vi "WHD_VEten_0.1.4.WS_BIDIR_Cal_05_03_2020.vi"() -> ()   [LabVIEW 2015]
uses:
  <vilib>/LabVIEW Targets/FPGA/cRIO/shared/nicrio_ModuleControls/nicrio_cRIO-9234_DataRatesRing2.ctl
  <vilib>/RTwatchdog.llb/Watchdog expiration actions.ctl
  <vilib>/userdefined/High Color/nirio_resource_hc.ctl
  <vilib>/Platform/TimedLoop/XDataNode/timing_clust.ctl
  <vilib>/Platform/TimedLoop/XDataNode/nitl_modes.ctl
  <vilib>/Platform/TimedLoop/XDataNode/wakeup.ctl
  <vilib>/Analysis/5stat.llb/RMS (DBL).vi
  <vilib>/FPGAPlugInAG/cRIO-9031/niLvFpga_Open_cRIO-9031.vi
  <vilib>/Utility/error.llb/Error Cluster From Error Code.vi
  <vilib>/rvi/errors/niLvFpgaAdjustHostInterfaceError.vi
  <vilib>/FPGAPlugInAG/cRIO-9031/niLvFpga_Run_cRIO-9031.vi
  <vilib>/rvi/interface/common/niFpgaWaitOnOcc.vi
  <vilib>/Utility/file.llb/Write Delimited Spreadsheet (string).vi
  <vilib>/FPGAPlugInAG/cRIO-9031/niLvFpga_Reset_cRIO-9031.vi
  <vilib>/measure/madcrms.llb/Basic Averaged DC-RMS for 1 Chan.vi
  <vilib>/measure/maspectr.llb/FFT Spectrum (Mag-Phase) for 1 Chan.vi
  <vilib>/Utility/config.llb/Write Key (Double).vi
  <vilib>/FPGAPlugInAG/cRIO-9031/niLvFpga_Close_cRIO-9031.vi
  <vilib>/rvi/interface/nirviOpenFPGA/nirviOpenFPGA.xnode
  FPGA Bitfiles/W_RDArabia_FPGATarget_FPGA8a2wsBIdirec_yJvL9yuTbZw.lvbitx
  <vilib>/rvi/interface/nirviReadWriteControl/nirviReadWriteControl.xnode
  <vilib>/rvi/interface/nirviMethod/nirviMethod.xnode
  <vilib>/platform/TimedLoop/XDataNode/XDataNode.xnode
  <vilib>/rvi/interface/nirviCloseFPGA/nirviCloseFPGA.xnode
  <vilib>/NI_Real-Time Target Support.lvlib
  <vilib>/rvi/errors/niLvFpgaMergeErrorWithErrorCode.vi
  AURA_Wheel/Json2Labv.lvlib
  AURA_Wheel/AuraWheelAPI/AuraWheel.lvlib
  NiFpgaLv.dll
  <vilib>/FPGAPlugInAG/cRIO-9031/niLvFpga_ConfigureFifo_cRIO-9031.vi
  <vilib>/FPGAPlugInAG/cRIO-9031/niLvFpga_StartFifo_cRIO-9031.vi
  <vilib>/FPGAPlugInAG/cRIO-9031/niLvFpga_ReadFifo_cRIO-9031.vi
  <vilib>/FPGAPlugInAG/cRIO-9031/niLvFpga_StopFifo_cRIO-9031.vi
  <vilib>/measure/NI_MAPro.lvlib
  <vilib>/Analysis/NI_AALPro.lvlib
  <vilib>/Analysis/NI_AALBase.lvlib
  <vilib>/Utility/config.llb/NI_LVConfig.lvlib
  <vilib>/Platform/TimedLoop/XDataNode/XDNodeRunTimeDep.lvlib
  Library/IF2_Reader/IF2_Reader.lvlib
panel:
  out "T fuera rango":bool
  out "Frequency":dbl[](array[numeric])
  out "Value to compare":dbl[](array[numeric])
  in  "Developer password":string
  out "Waveform Graph":waveform(sgl)[](graph)
  out "min":dbl[](array[numeric])
  out "max":dbl[](array[numeric])
  out "median":dbl[](array[numeric])
  out "mean":dbl[](array[numeric])
  in  "Accelerometer":i32=1 min=1 max=8
  out "Low cutoff freq":dbl
  out "noise_range":dbl
  out "Numeric":i32
  out "Calibration parameter":dbl
  out "Accel.detected":i32
  out "Mean\nfrequency":dbl format="%0.2f"
  out "Nº meas":i32
  out "Array":i32[](array[numeric])
  out "sorted array":i32[](array[numeric])
  out "Array 3":i32[](array[numeric])
  out "max value":i32
  out "max index(es)":i32
  out "element":i32
  out "size(s) 3":i32
  out "size(s)":i32[](array[numeric])
  out "Valid\nindex":i32[](array[numeric])
  out "Acquiring time":dbl
  out "Inicio pasada 2":timestamp
  out "calibration log":path
  out "date/time string 2":string
  out "Folder":path
  in  "Developer commad":string
  out "Save calibration":bool
  out "Pattern amplitude (g)":dbl=1.02
  out "Pattern frequency (Hz)":dbl=159.2
  out "Report":string
  out "AURA wheel test":bool
  out "LOG.txt":path
  out "Report_AURA":string
  out "error FPGA":errorcluster
  out "error AURA":errorcluster
  out "error manipulacion archivos":errorcluster
  out "Response headers":string
  out "Max RMS Ruedas":dbl[][](array[numeric])
  out "TAGs LR6":string[](array[string])
  out "TAGs HEX":string[](array[string])
  out "Parar":bool
  out "result":bool
  out "TAGs":string[](array[string])
  out "Temperatura (ºC)":dbl
  out "V (m/s)":dbl
  out "Digital?":bool=TRUE
  out "Watchdog config":T1={"reset"=FALSE, "occurrence"=FALSE, "trigger protocol"=enum."active high", "trigger line"=enum."none", "disable watchdog on VI exit"=TRUE}
  out "Tiempo de adquisicion":dbl=10.0
  out "Adquirir":bool
  out "Nº Ruedas 1":i32
  out "NºRuedas 2":i32
  out "Disco Duro Disponible (bytes)":i64
  out "Buffer Overflow":bool
  out "Buffer Underflow":bool
  out "Archivo\nvalido?":bool
  out "Número de ejes detectados":i32
  out "Ejes_convoy":i32
  out "Tiempo de paso (s)":dbl
  out "created path":path
  out "Nombre de archivo":path[](array[path])
  out "LR6 IP address":string="192.168.106.94"
  out "Port LR6":u16=2001
  out "Frecuencia de muestreo (Hz)":dbl=25600.0
  out "Escaneos de la FIFO por canal":u32=5000
  out "Tiempo extra al detector de paso (s)":dbl=1.0
  out "dt RMS":dbl=256.0
  out "Frecuencia de muestreo y módulo CRIO":T2=2 items=["51.200 kS/s (NI 9234)"=1, "25.600 kS/s (NI 9234)"=2, "17.067 kS/s (NI 9234)"=3, "12.800 kS/s (NI 9234)"=4, "10.240 kS/s (NI 9234)"=5, "8.533 kS/s (NI 9234)"=6, "7.314 kS/s (NI 9234)"=7, "6.400 kS/s (NI 9234)"=8, "5.689 kS/s (NI 9234)"=9, "5.120 kS/s (NI 9234)"=10, "4.654 kS/s (NI 9234)"=11, "4.267 kS/s (NI 9234)"=12, "3.938 kS/s (NI 9234)"=13, "3.657 kS/s (NI 9234)"=14, "3.413 kS/s (NI 9234)"=15, "3.200 kS/s (NI 9234)"=16, "3.012 kS/s (NI 9234)"=17, "2.845 kS/s (NI 9234)"=18, "2.695 kS/s (NI 9234)"=19, "2.560 kS/s (NI 9234)"=20, "2.438 kS/s (NI 9234)"=21, "2.328 kS/s (NI 9234)"=22, "2.226 kS/s (NI 9234)"=23, "2.133 kS/s (NI 9234)"=24, "2.048 kS/s (NI 9234)"=25, "1.969 kS/s (NI 9234)"=26, "1.896 kS/s (NI 9234)"=27, "1.829 kS/s (NI 9234)"=28, "1.765 kS/s (NI 9234)"=29, "1.707 kS/s (NI 9234)"=30, "1.652 kS/s (NI 9234)"=31]
  out "Puerto RFID":u16=2189
  out "IP RFID":string="192.168.106.99"
  out "Offset_rueda WS 2":fxp<+/-,24,-4>=0.004999998956918716 format="%.27g"
  out "Count(mSec)":u32=2
  out "RFID NEM on?":bool
  out "RFID LR6 on?":bool
  out "Canal cero WS1?":bool
  out "Canal cero WS2":bool
  in  "Calibration":bool
  out "Direccion 0?":bool
  out "Boton Adquirir?":bool
  out "RuedaDetectada2?":bool=TRUE
  out "RuedaDetectada1?":bool=TRUE
  out "Timeout ruedas":dbl
  out "Borrar archivos\nadquisicion con error":bool
  out "Able watchdog?":bool
  out "Reset watchdog?":bool
  out "Leer config RFID NEM":bool
  out "bytes to read":i32
  out "DeviceAddress":u8
  out "timeout ms (60000)":i32
  out "Max archivos":u32=2
  out "Bytes libre despues de borrar":u32=2
  out "Bytes min libre":u32=2
  out "Nº de acelerómetros":i32
  out "Nº inductivos":i32
  out "Offset_rueda WS 1":fxp<+/-,24,-4>=0.004999998956918716 format="%.27g"
  out "TAGs_AURAwheel":string[][](array[string])
  out "Plataformas?":bool
  out "Nº Ejes":i32[](array[numeric])
  out "Nº UTs":i32
  out "it-read-LR6":i32[](array[numeric])
  out "it-LR6":i32
  out "RFID_LR6_Error":errorcluster
  out "Series_flota":string[](array[string])
  out "Tabla_flota":string[][](array[string])
  out "Puntos medios de las ventanas":dbl[][](array[numeric])
  out "configuration file path":path=path "c:/Parametros.cfg"
  out "IP synchr":string
  out "data":cluster{"status":string}
  out "confRFID":path=path "c:/RFID/TAGS.csv"
  out "TAGS leidos":path=path "c:/RFID/TAGS.csv"
  out "Use Aura?":bool
  out "Parametros AuraWheel":string[](array[string])
  out "Parámetros acelerómetros":dbl[](array[numeric])
  out "Fin":bool
  out "Contador":i32=1
  out "Path LOG":path=path "c:/TEST"
  out "Fallo fotocelula":bool
  out "Path_Borrar":path=path "c:/Trenes"
  out "Longitud de la unidad":dbl
  out "Aviso no detección":string
  out "Time to Acquire Block (ms)":i32
  out "Distancia de acelerómetros":dbl[](array[numeric])
  out "Block Size":u32
  out "Distancias generales":dbl[](array[numeric])
  out "Reset del controlador":bool
  out "Parar la aplicación":bool
  out "date/time string":string
  out "Timeout ruedas":bool
  out "Tiempo":dbl
  out "Inicio pasada":timestamp
  out "Ultimo TEST":timestamp
  out "Fuente":bool=TRUE
  out "DC OK":string
  out "Aviso temperatura":string
  out "connection ID":refnum<k5>
  # "Calibration - Noise analysis"
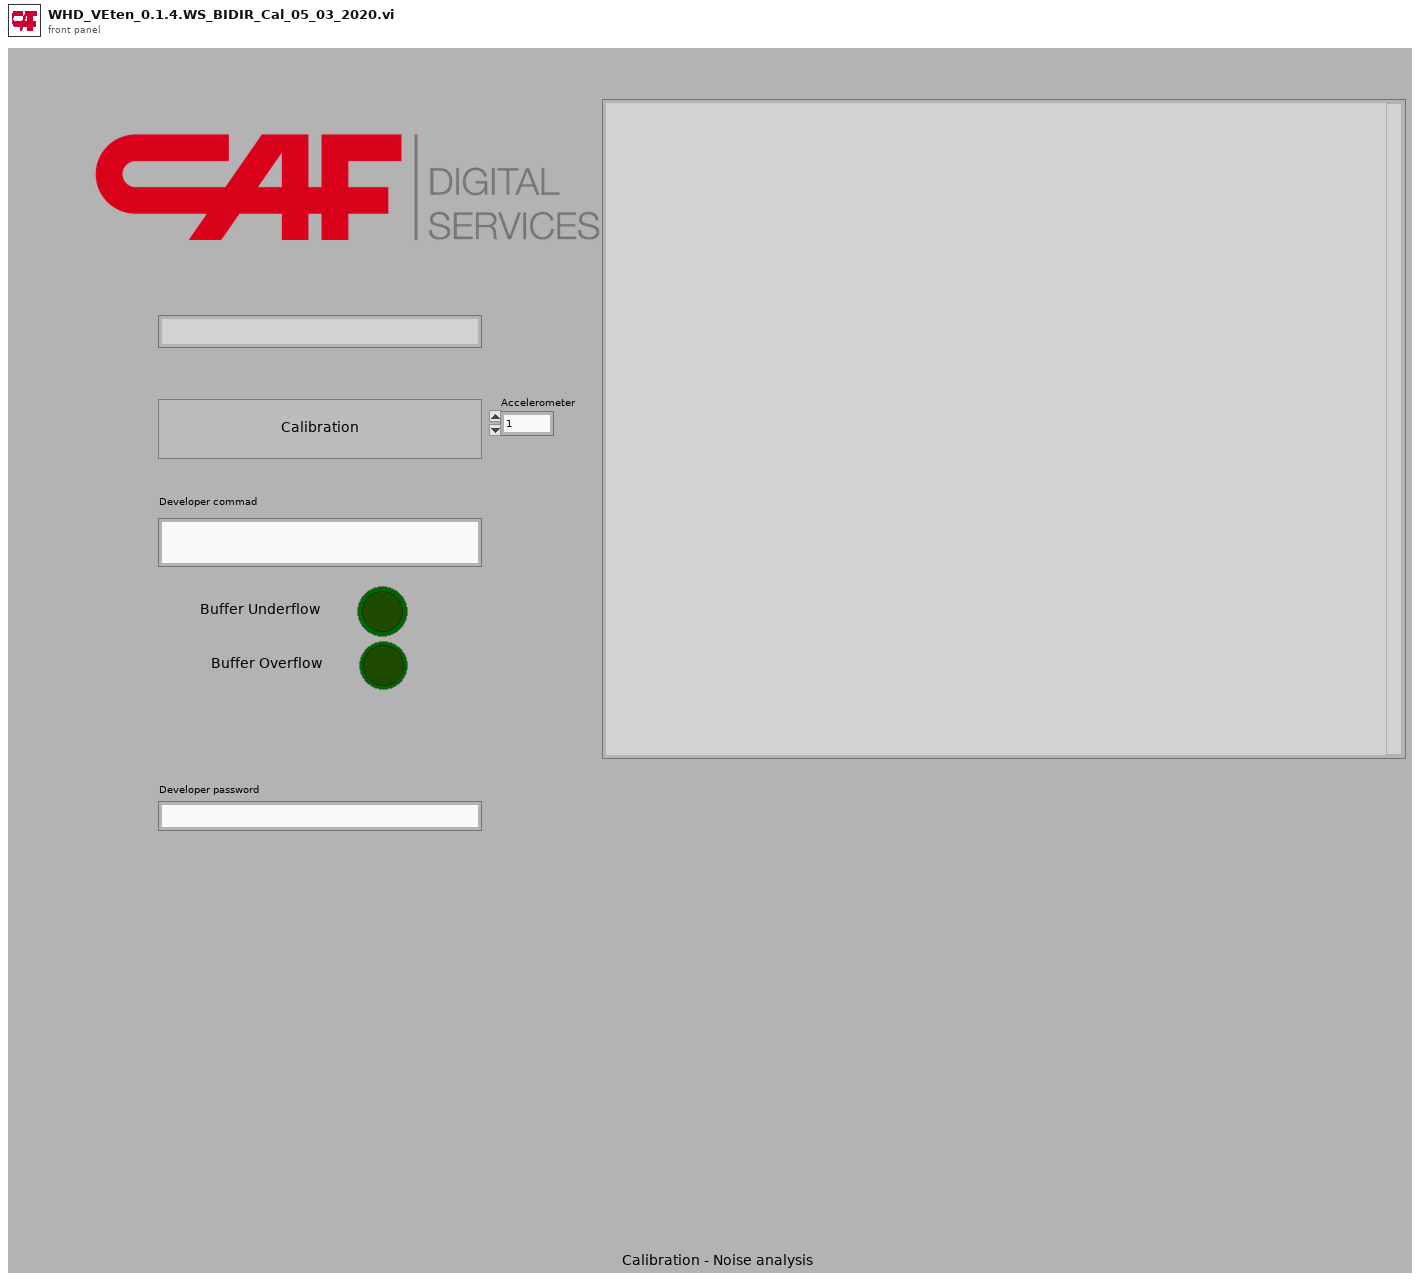
[diagram p1: front panel]
types:
  T1 = typedef "Watchdog expiration actions.ctl" = cluster{"reset":bool, "occurrence":bool, "trigger protocol":enum16{"active high", "active low", "open collector"}, "trigger line":enum16{"none", "line 0", "line 1", "line 2", "line 3", "line 4", "line 5", "line 6", "line 7", "SMB line 0"}, "disable watchdog on VI exit":bool}
  T2 = typedef "nicrio_cRIO-9234_DataRatesRing2.ctl" = u8
  T3 = typedef "nirio_resource_hc.ctl" = tag
  T4 = enum16{"open", "replace", "create", "open or create", "replace or create", "replace or create with confirmation"}
  T5 = enum16{"big-endian, network order", "native, host order", "little-endian"}
  T6 = typedef "XDNodeRunTimeDep.lvlib/timing_clust.ctl" = cluster{"Expected End [f-1]":u64, "Actual End [f-1]":u64, "Finished Late? [f-1]":bool, "Expected End [i-1]":u64, "Actual End [i-1]":u64, "Finished Late? [i-1]":bool, "Expected Start [i]":u64, "Actual Start [i]":u64, "Expected Start [f]":u64, "Actual Start [f]":u64, "Source Name":string, "Structure Name":string, "Period":i64, "Deadline":i64, "Offset":i64, "Start":i64, "Priority":i32, "Timeout":i32, "Mode":T7, "Wakeup Reason":T8, "Error":errorcluster, "Source Type":string, "Secondary Source Type":string, "Global End Time":u64, "Global Start Time":u64, "Frame Duration":u64, "Iteration Duration":u64, "Assigned CPU":i32, "I/O Scan Engine Mode":u32}
  T7 = typedef "XDNodeRunTimeDep.lvlib/nitl_modes.ctl" = enum32{"No Change", "Process missed periods, maintain original phase", "Discard missed periods, maintain original phase", "Process missed periods, ignore original phase", "Discard missed periods, ignore original phase"}
  T8 = typedef "XDNodeRunTimeDep.lvlib/wakeup.ctl" = enum32{"Normal", "Aborted", "Asynchronous wakeup", "Timing source error", "Timed loop error", "Timeout"}
  T9 = cluster{"error IO":errorcluster, bool[], u32[], string[], dbl[]}
  T10 = cluster{"error out":errorcluster, dbl[], "Normalized Tags":string[], "Direccion 0?":bool}
  T11 = cluster{"g_ts":dbl, "p_sp":dbl, "p_tp":dbl, "p_tg":cluster{"tg_n":dbl, "tg_t":string}[], "p_ax":cluster{"ax_n":dbl, "ax_sp":dbl, "ax_wh":cluster{"wh_p":dbl, "wh_a1":dbl, "wh_a2":dbl, "wh_a3":dbl, "wh_a4":dbl}[]}[]}
  T12 = typedef "NI_LVConfig.lvlib/Config Data RefNum.ctl" = refnum<k1>
  T13 = cluster{"IP":string, "Port":u16, "ReaderConfigFile":path, "ROspecConfigFile":path}
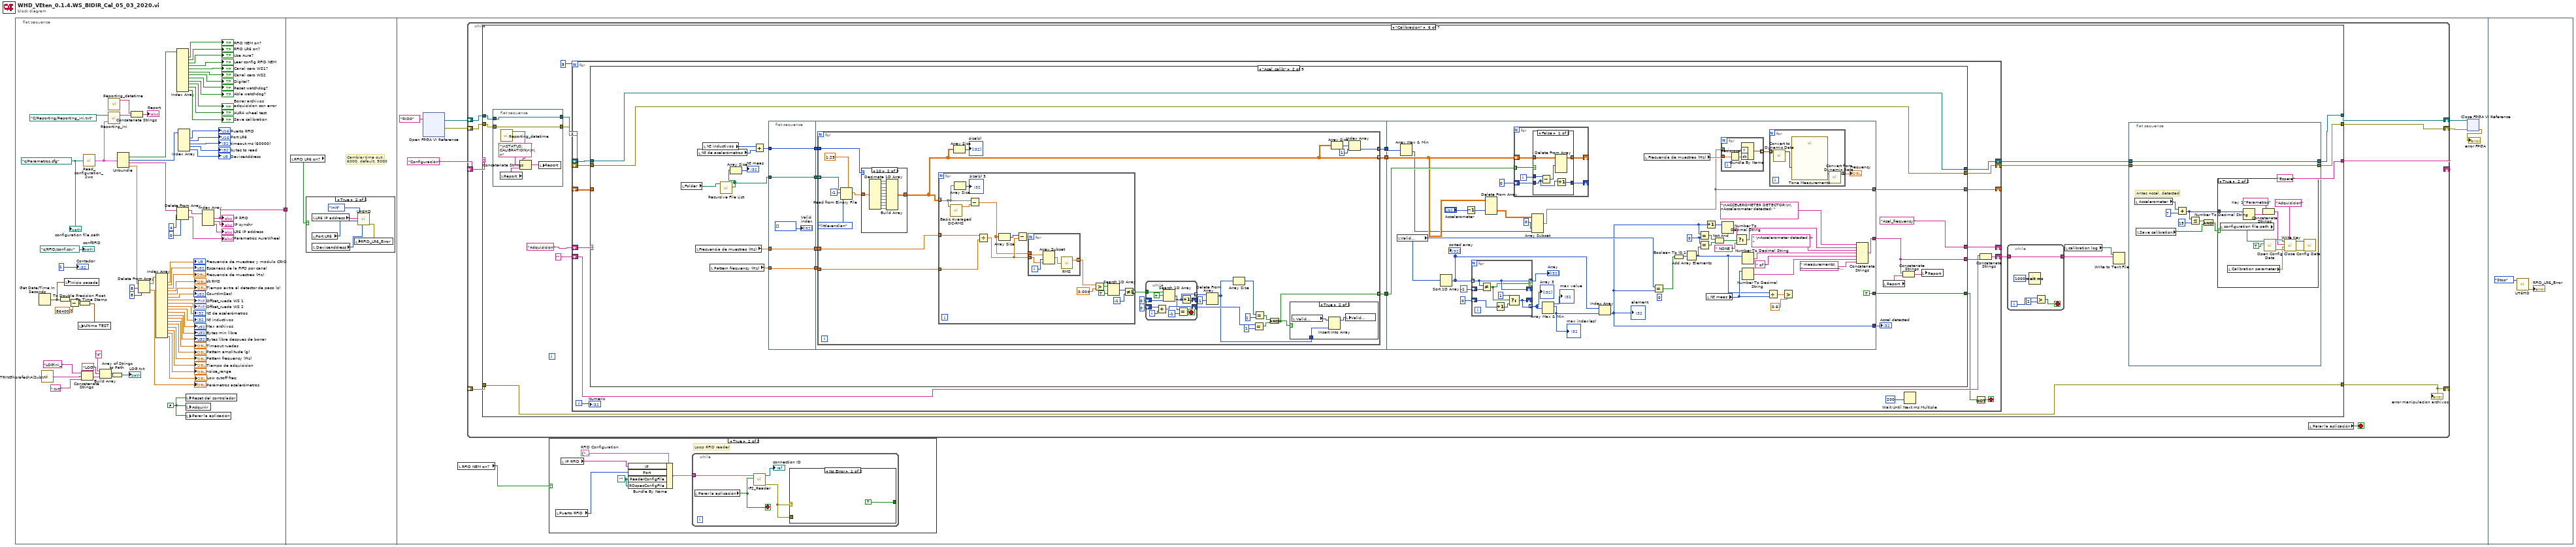
[diagram p0: block diagram]
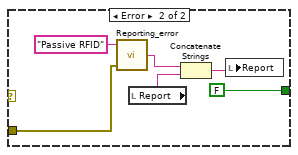
[diagram p4: hidden frame]
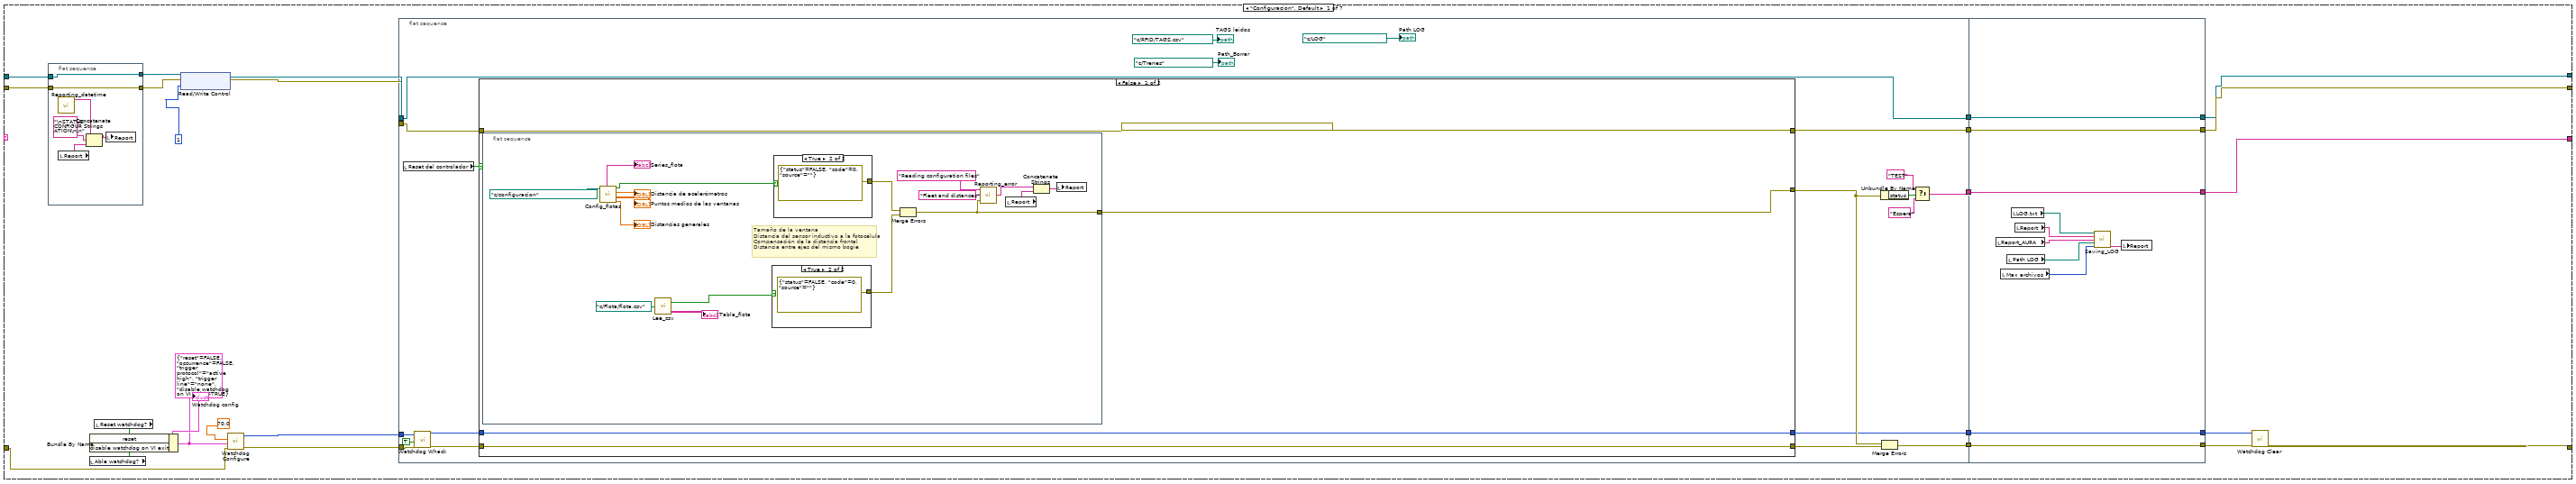
[diagram p5: hidden frame]
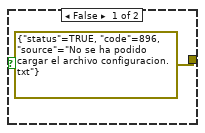
[diagram p6: hidden frame]
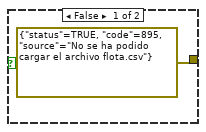
[diagram p7: hidden frame]
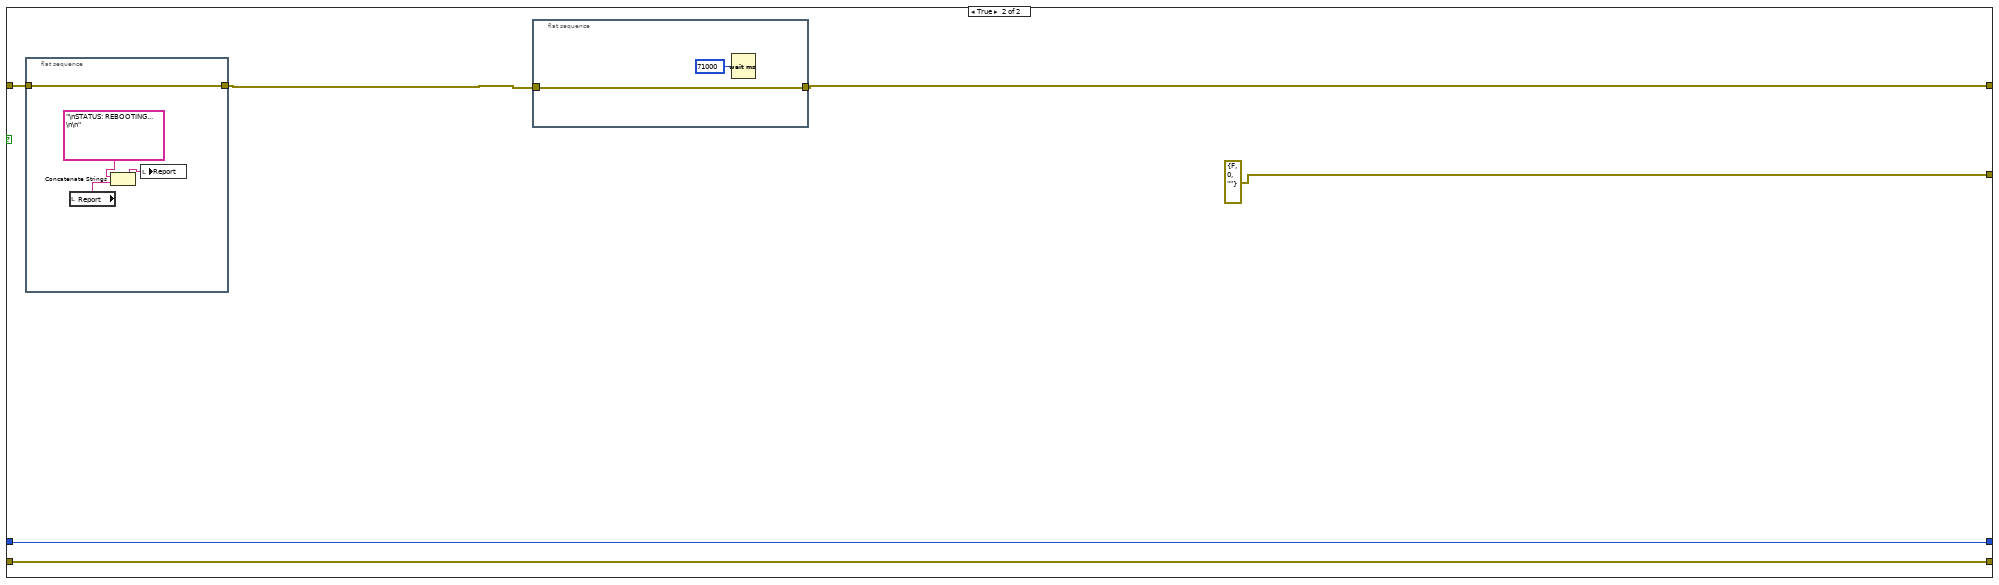
[diagram p8: hidden frame]
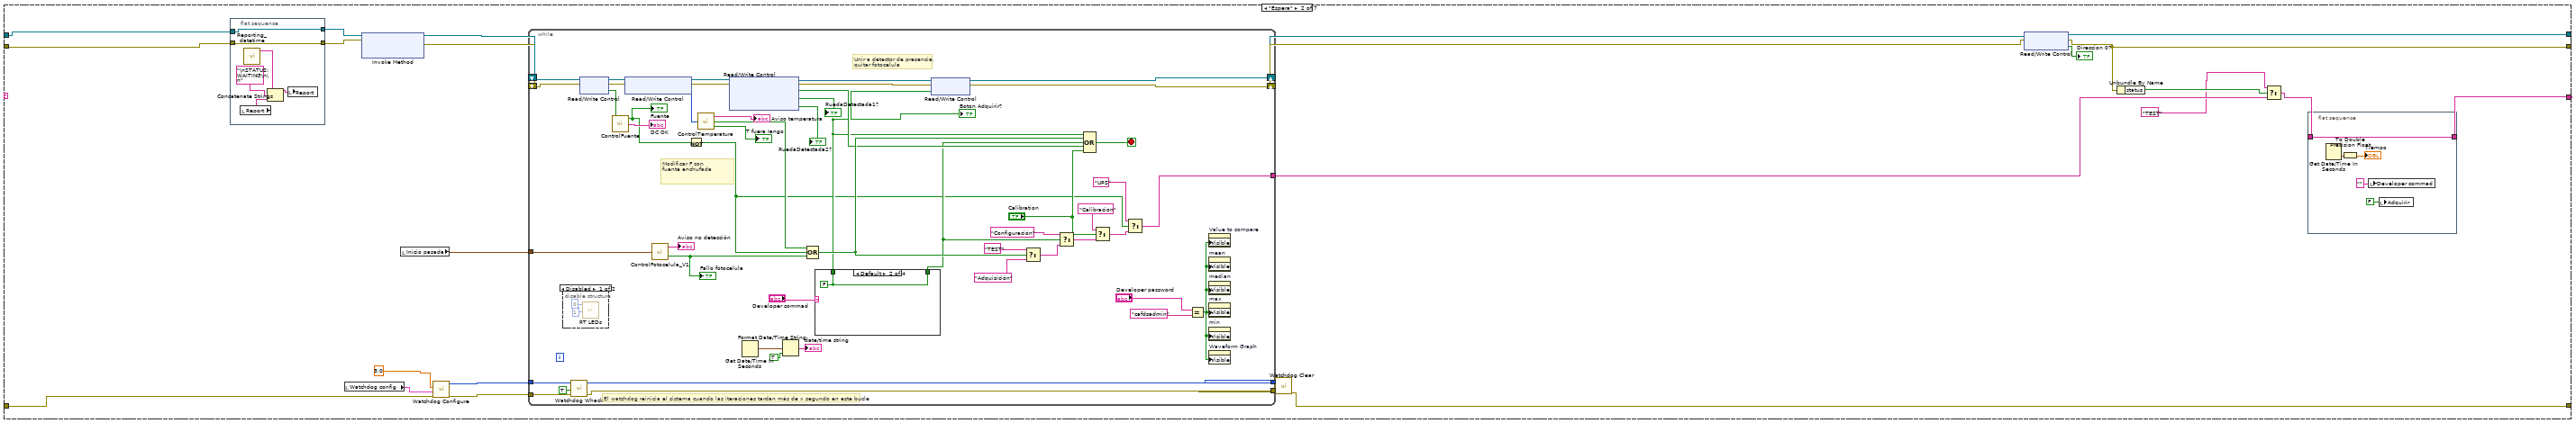
[diagram p9: hidden frame]
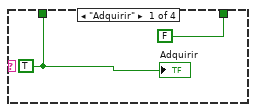
[diagram p10: hidden frame]
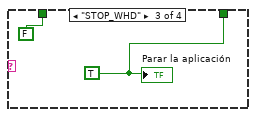
[diagram p11: hidden frame]
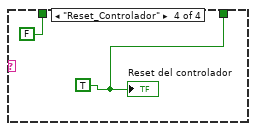
[diagram p12: hidden frame]
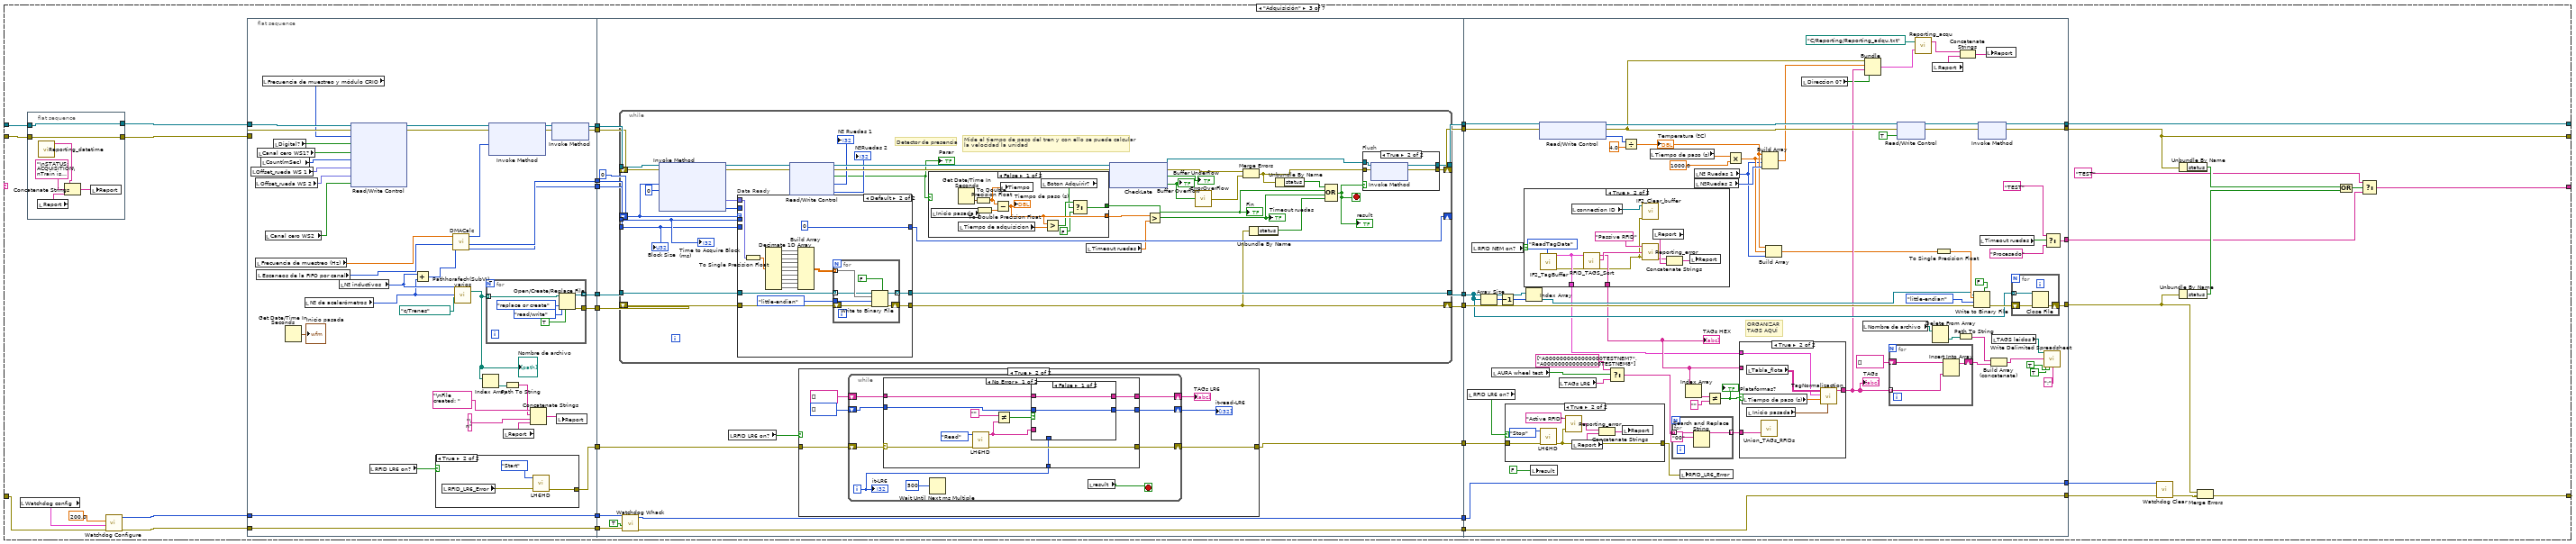
[diagram p14: hidden frame]
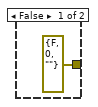
[diagram p15: hidden frame]
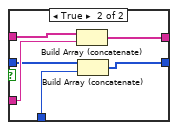
[diagram p17: hidden frame]
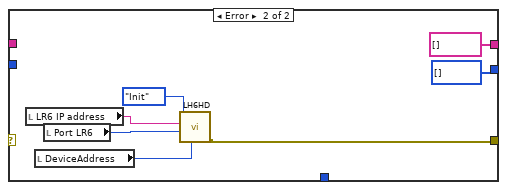
[diagram p18: hidden frame]
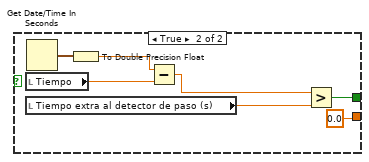
[diagram p19: hidden frame]
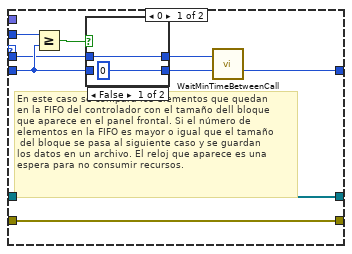
[diagram p20: hidden frame]
diagram:
  n1 = flat-sequence {
    tunnel: [w4] -> w1
    tunnel: w1 -> [_]
    frame #0 {
      w5 = FALSE ("Reset del controlador")
      w66 = path "c:/Parametros.cfg" ("configuration file path")
      n2 = Get Date/Time In Seconds() -> (seconds since 1Jan1904=w71:timestamp)
      n3 = call "STRINGhorafechA(SubVI).vi"() -> ("STRINGhora_fecha"=w16:string)
      n4 = To Double Precision Float(number=w71) -> (double precision float=w73:dbl)
      n5 = local write "Inicio pasada"(w71) -> ()
      n6 = Subtract(x=w73, y=86400.0) -> (x-y=w72:dbl)
      n7 = To Time Stamp(1:w72) -> (0:w70:timestamp)
      n8 = local write "Ultimo TEST"(w70) -> ()
      n9 = Concatenate Strings("LOGini_" ("string"), w16, ".txt" ("string")) -> (w18:string)
      n10 = call "Read_configuration_2ws.vi"("configuration file path"=w66) -> ("output cluster"=w22:T9)
      n11 = Build Array("c", "LOG" ("element"), w18) -> (w15:string[])
      n12 = call "Reporting_ini.vi"("Configuration cluster"=w22, "address repoting"=path "C:/Reporting/Reporting_ini.txt" ("file (use dialog)")) -> ("Reporting"=w21:string)  [unwired: 1 in]
      n13 = call "Reporting_datetime.vi"() -> ("String"=w19:string)  [unwired: 11 in]
      n14 = Array of Strings to Path(0:w15) -> (2:→"LOG.txt":path)  [unwired: 1 out]
      n15 = Unbundle(w22) -> (w69:bool[], w68:u32[], w61:string[], w65:dbl[])  [unwired: 1 out]
      n16 = Concatenate Strings(w19, w21) -> (→"Report":string)
      n17 = Delete From Array(array=w65, length=8, index=8) -> (deleted portion=→"Parámetros acelerómetros":dbl[], array with subset deleted=w64:dbl[])
      n18 = Index Array(array=w64) -> (element #1=→"Frecuencia de muestreo y módulo CRIO":dbl, element #2=→"Escaneos de la FIFO por canal":dbl, element #3=→"Frecuencia de muestreo (Hz)":dbl, element #4=→"dt RMS":dbl, element #5=→"Tiempo extra al detector de paso (s)":dbl, element #6=→"Count(mSec)":dbl, element #7=→"Offset_rueda WS 1":dbl, element #8=→"Offset_rueda WS 2":dbl, element #9=→"Nº de acelerómetros":dbl, element #10=→"Nº inductivos":dbl, element #11=→"Max archivos":dbl, element #12=→"Bytes min libre":dbl, element #13=→"Bytes libre despues de borrar":dbl, element #14=→"Timeout ruedas":dbl, element #15=→"Pattern amplitude (g)":dbl, element #16=→"Pattern frequency (Hz)":dbl, element #17=→"Tiempo de adquisicion":dbl, element #18=→"noise_range":dbl, element #19=→"Low cutoff freq":dbl)  [unwired: 19 in]
      n19 = Index Array(array=w69) -> (element #1=→"RFID NEM on?":bool, element #2=→"RFID LR6 on?":bool, element #3=→"Use Aura?":bool, element #4=→"Leer config RFID NEM":bool, element #5=→"Canal cero WS1?":bool, element #6=→"Canal cero WS2":bool, element #7=→"Digital?":bool, element #8=→"Reset watchdog?":bool, element #9=→"Able watchdog?":bool, element #10=→"Borrar archivos\nadquisicion con error":bool, element #11=→"AURA wheel test":bool, element #12=→"Save calibration":bool)  [unwired: 12 in]
      n20 = Delete From Array(array=w61, length=4, index=0) -> (deleted portion=→"Parametros AuraWheel":string[], array with subset deleted=w60:string[])
      n21 = Index Array(array=w68) -> (element #1=→"Puerto RFID":u32, element #2=→"Port LR6":u32, element #3=→"timeout ms (60000)":u32, element #4=→"bytes to read":u32, element #5=→"DeviceAddress":u32)  [unwired: 5 in]
      n22 = local write "Reset del controlador"(w5) -> ()
      n23 = local write "Adquirir"(w5) -> ()
      n24 = local write "Parar la aplicación"(w5) -> ()
      n25 = Index Array(array=w60) -> (element #1=w4:string, element #2=→"IP synchr":string, element #3=→"LR6 IP address":string)  [unwired: 3 in]
      "IP RFID" <- w4
      "Contador" <- 1
      "confRFID" <- path "c:/RFID/conf.csv" ("file path (use dialog)")
      "configuration file path" <- w66
    }
    frame #1 {
      # "Cambiar time out:\n6000, default, 5000"
      n26 = local read "RFID LR6 on?"() -> (w75:bool)
      n27 = case shown="True" w75 {
        frame False {
        }
        frame True {
          n28 = local read "LR6 IP address"() -> (w76:string)
          n29 = local read "Port LR6"() -> (w77:u16)
          n30 = local read "DeviceAddress"() -> (w78:u8)
          n31 = call "LH6HD.vi"("DeviceAddress"=w78, "Reader Port"=w77, "IP Address"=w76, "Action"=enum16{"Init", "Start", "Read", "Stop", "Exit"}."Init") -> ("error out"=w80:errorcluster)  [unwired: 6 in, 1 out]
          n32 = local write "RFID_LR6_Error"(w80) -> ()
        }
      }
    }
    frame #2 {
      n33 = xnode "Open FPGA VI Reference"("resource name"=T3 "RIO0") -> ("FPGA VI Reference Out"=w88:refnum<k20>, "error out"=w87:errorcluster)  [unwired: 1 in]
      n34 = local read "RFID NEM on?"() -> (w81:bool)
      n35 = while {
        shift-right: [w105] -> _
        shift-left: "Configuración" -> [w113]
        shift-right: [w107] -> w84
        shift-left: w88 -> [w112]
        shift-right: [w106] -> w83
        shift-left: w87 -> [w111]
        shift-right: [w110] -> _
        shift-left: _ -> [w109]
        stop <- w108 stop-if-true
        n36 = case shown="\"Calibracion\"" w113 {
          tunnel: [w128 w231 w326 w676 w924 "Espera" "Espera" ("t")] -> w105
          tunnel: [w138 w219 w340 w665 w923 w992 w1791] -> w107
          tunnel: [w139 w218 w341 w663 w922 w990 w1790] -> w106
          tunnel: w112 -> [w122 w217 w312 w666 w923 w1002 w1793]
          tunnel: w111 -> [w121 w216 w311 w664 w915 w1001 w1792]
          tunnel: [w135 w225 w338 w661 w914 w991 w1788] -> w110
          tunnel: w109 -> [w127 w230 w322 w675 w911 w991 w1788]
          frame "Configuración", Default {
            n37 = flat-sequence {
              tunnel: w122 -> [w145]
              tunnel: w121 -> [w144]
              tunnel: [w145] -> w120
              tunnel: [w144] -> w119
              frame #0 {
                n38 = call "Reporting_datetime.vi"() -> ("String"=w140:string)  [unwired: 11 in]
                n39 = local read "Report"() -> (w141:string)
                n40 = Concatenate Strings(w140, "\nSTATUS: CONFIGURATION\n\n", w141) -> (w143:string)
                n41 = local write "Report"(w143) -> ()
              }
            }
            n42 = local read "Able watchdog?"() -> (w132:bool)
            n43 = local read "Reset watchdog?"() -> (w133:bool)
            n44 = Bundle By Name(cluster=T1 {"reset"=FALSE, "occurrence"=FALSE, "trigger protocol"=enum."active high", "trigger line"=enum."none", "disable watchdog on VI exit"=TRUE} ("expiration actions"), "reset"=w133, "disable watchdog on VI exit"=w132) -> (w126:T1)
            "Watchdog config" <- w126
            n45 = xnode "Read/Write Control"("FPGA VI Reference In"=w120, "error in"=w119, "Cycles to Filter"=u16 1) -> ("FPGA VI Reference Out"=w131:refnum<k20>, "error out"=w130:errorcluster)
            n46 = call <vilib>:"Watchdog Configure.vi"("error in (no error)"=w127, "expiration actions"=w126, "timeout (1 sec)"=70.0) -> ("error out"=w123:errorcluster, "watchdogID"=w124:u64)  [unwired: 1 in, 2 out]
            n47 = flat-sequence {
              tunnel: w131 -> [w157]
              tunnel: w130 -> [w154]
              tunnel: w124 -> [w147]
              tunnel: w123 -> [w146]
              tunnel: [w156] -> w118
              tunnel: [w164] -> w117
              tunnel: [w157] -> w116
              tunnel: [w159] -> w115
              tunnel: [w151] -> w114
              tunnel: [w209] -> w137
              tunnel: [w210] -> w136
              tunnel: [w211] -> w138
              tunnel: [w212] -> w128
              tunnel: [w213] -> w139
              tunnel: w118 -> [w213]
              tunnel: w117 -> [w212]
              tunnel: w116 -> [w211]
              tunnel: w115 -> [w210]
              tunnel: w114 -> [w209]
              frame #0 {
                n48 = local read "Reset del controlador"() -> (w153:bool)
                n49 = call <vilib>:"Watchdog Whack.vi"("error in (no error)"=w146, "reset watchdog after expire? (F)"=TRUE, "watchdogID in"=w147) -> ("error out"=w149:errorcluster, "watchdogID out"=w150:u64)  [unwired: 2 in, 1 out]
                n50 = case shown="False" w153 {
                  tunnel: w154 -> [w169 w192]
                  tunnel: [w169 w195] -> w156
                  tunnel: [w166 errorcluster {"status"=FALSE, "code"=0, "source"=""} ("error IO")] -> w155
                  tunnel: [w168 w194] -> w151
                  tunnel: w150 -> [w168 w194]
                  tunnel: w149 -> [w167 w193]
                  tunnel: [w167 w193] -> w148
                  frame False {
                    n51 = flat-sequence {
                      tunnel: [w170] -> w166
                      frame #0 {
                        # "Tamaño de la ventana\nDistancia del sensor inductivo a la fotocélula\nCompensación de la distancia frontal\nDistancia entre ejes del mismo bogie"
                        n52 = call "Config_flotas.vi"("file path (dialog if empty)"=path "c:/configuracion") -> ("Distancias generales"=→"Distancias generales":dbl[], "Puntos medios de las ventanas"=→"Puntos medios de las ventanas":dbl[][], "Distancia de acelerómetros"=→"Distancia de acelerómetros":dbl[], "Distacias y medidas de dispositivos"=w183:bool, "Series_flota"=→"Series_flota":string[])  [unwired: 3 in]
                        n53 = call "Lee_csv.vi"("Path"=path "c:/Flota/flota.csv") -> ("Tabla_flota"=→"Tabla_flota":string[][], "Lectura_OK?"=w180:bool)
                        n54 = case shown="True" w180 {
                          tunnel: [errorcluster {"status"=TRUE, "code"=895, "source"="No se ha podido cargar el archivo flota.csv"} ("error out") errorcluster {"status"=FALSE, "code"=0, "source"=""} ("error out")] -> w184
                          frame False {
                          }
                          frame True {
                          }
                        }
                        n55 = case shown="True" w183 {
                          tunnel: [errorcluster {"status"=TRUE, "code"=896, "source"="No se ha podido cargar el archivo configuracion.txt"} ("error out") errorcluster {"status"=FALSE, "code"=0, "source"=""} ("error out")] -> w185
                          frame False {
                          }
                          frame True {
                          }
                        }
                        n56 = Merge Errors(w185, w184) -> (w170:errorcluster)
                        n57 = call "Reporting_error.vi"("error out 2"=w170, "Concept explanation"="Fleet and distances", "Concept"="Reading configuration files") -> ("Reporting"=w172:string)
                        n58 = local read "Report"() -> (w171:string)
                        n59 = Concatenate Strings(w172, w171) -> (w173:string)
                        n60 = local write "Report"(w173) -> ()
                      }
                    }
                  }
                  frame True {
                    n61 = flat-sequence {
                      tunnel: w192 -> [w200]
                      tunnel: [w200] -> w191
                      frame #0 {
                        n62 = local read "Report"() -> (w199:string)
                        n63 = Concatenate Strings("\nSTATUS: REBOOTING...\n\n", w199) -> (w197:string)
                        n64 = local write "Report"(w197) -> ()
                      }
                    }
                    n65 = flat-sequence {
                      tunnel: [w202] -> w195
                      tunnel: w191 -> [w202]
                      frame #0 {
                        n66 = Wait (ms)(milliseconds to wait=u32 71000) -> ()  [unwired: 1 out]
                      }
                    }
                  }
                }
                n67 = Unbundle By Name(w155) -> ("status"=w165:bool)
                n68 = Merge Errors(w155, w148) -> (w159:errorcluster)
                n69 = Select(t="TEST", s=w165, f="Espera") -> (s? t:f=w164:string)
                "Path_Borrar" <- path "c:/Trenes" ("file path (use dialog)")
                "Path LOG" <- path "c:/LOG" ("file path (use dialog)")
                "TAGS leidos" <- path "c:/RFID/TAGS.csv" ("file path (use dialog)")
              }
              frame #1 {
                n70 = local read "Report_AURA"() -> (w206:string)
                n71 = local read "Max archivos"() -> (w207:u32)
                n72 = local read "Path LOG"() -> (w208:path)
                n73 = local read "LOG.txt"() -> (w203:path)
                n74 = local read "Report"() -> (w205:string)
                n75 = call "Saving_LOG.vi"("Path"=w203, "Report"=w205, "Report AURA"=w206, "Path Carpeta"=w208, "Nº Archivos Max"=w207) -> ("Report"=w204:string)  [unwired: 9 in, 1 out]
                n76 = local write "Report"(w204) -> ()
              }
            }
            n77 = call <vilib>:"Watchdog Clear.vi"("error in (no error)"=w136, "watchdogID in"=w137) -> ("error out"=w135:errorcluster)  [unwired: 5 in]
          }
          frame "Espera" {
            n78 = flat-sequence {
              tunnel: w217 -> [w244]
              tunnel: w216 -> [w243]
              tunnel: [w244] -> w215
              tunnel: [w243] -> w214
              frame #0 {
                n79 = local read "Report"() -> (w240:string)
                n80 = call "Reporting_datetime.vi"() -> ("String"=w239:string)  [unwired: 11 in]
                n81 = Concatenate Strings(w239, "\nSTATUS: WAITING\n\n", w240) -> (w242:string)
                n82 = local write "Report"(w242) -> ()
              }
            }
            n83 = local read "Watchdog config"() -> (w224:T1)
            n84 = xnode "Invoke Method"("FPGA VI Reference In"=w215, "error in"=w214) -> ("FPGA VI Reference Out"=w234:refnum<k20>, "error out"=w233:errorcluster)  [unwired: 1 in]
            n85 = local read "Inicio pasada"() -> (w238:timestamp)
            n86 = call <vilib>:"Watchdog Configure.vi"("error in (no error)"=w230, "expiration actions"=w224, "timeout (1 sec)"=3.0) -> ("error out"=w229:errorcluster, "watchdogID"=w228:u64)  [unwired: 1 in, 2 out]
            n87 = while {
              tunnel: [w255] -> w237
              shift-right: [w271] -> w220
              shift-left: w234 -> [w279]
              shift-right: [w270] -> w221
              shift-left: w233 -> [w278]
              tunnel: w238 -> [w282]
              tunnel: w229 -> [w268]
              tunnel: w228 -> [w269]
              tunnel: [w267] -> w227
              tunnel: [w266] -> w226
              stop <- w261 stop-if-true
              # "Modificar F con\nfuente enchufada"
              # "Unir a detector de presencia,\nquitar fotocelula"
              # "El watchdog reinicia el sistema cuando las iteraciones tardan más de x segundo en este bucle"
              n88 = disable-structure shown="Disabled" {
                frame Disabled {
                  n89 = call <vilib>:"RT LEDs.vi"("State"=1, "LED Num"=0) -> ()  [unwired: 1 in, 5 out]
                }
                frame Enabled {
                }
              }
              n90 = call <vilib>:"Watchdog Whack.vi"("error in (no error)"=w268, "reset watchdog after expire? (F)"=TRUE, "watchdogID in"=w269) -> ("error out"=w266:errorcluster, "watchdogID out"=w267:u64)  [unwired: 2 in, 1 out]
              n91 = xnode "Read/Write Control"("FPGA VI Reference In"=w279, "error in"=w278) -> ("FPGA VI Reference Out"=w291:refnum<k20>, "error out"=w290:errorcluster, "DC OK"=w295:bool)
              n92 = call "ControlFuente.vi"("DC OK 3"=w295) -> ("DC OK 2"=w257:bool, "DC OK"=→"DC OK":string)  [unwired: 1 out]
              "Fuente" <- w257
              n93 = xnode "Read/Write Control"("FPGA VI Reference In"=w291, "error in"=w290) -> ("FPGA VI Reference Out"=w286:refnum<k20>, "error out"=w285:errorcluster, "Chassis Temperature"=w293:i16)
              n94 = call "ControlFotocelula_V1.vi"("Tiempo de entrada a espera"=w282) -> ("Aviso no detección"=→"Aviso no detección":string, "Boolean"=w283:bool)
              "Fallo fotocelula" <- w283
              n95 = Not(x=w257) -> (.not. x?=w253:bool)
              n96 = call "ControlTemperatura.vi"("Chassis Temperature"=w293) -> ("Aviso temperatura"=→"Aviso temperatura":string, "Boolean"=w287:bool, "T fuera rango"=→"T fuera rango":bool)
              n97 = xnode "Read/Write Control"("FPGA VI Reference In"=w286, "error in"=w285) -> ("FPGA VI Reference Out"=w281:refnum<k20>, "error out"=w280:errorcluster, "Detector de presencia"=w274:bool, "RuedaDetectada1?"=→"RuedaDetectada1?":bool, "RuedaDetectada2?"=→"RuedaDetectada2?":bool)
              n98 = Get Date/Time In Seconds() -> (seconds since 1Jan1904=w276:timestamp)
              n99 = Format Date/Time String(seconds (now)=w276, UTC format=TRUE) -> (date/time string=→"date/time string":string)  [unwired: 1 in]
              n100 = Compound Arithmetic op=OR(w287, w253, w283) -> (w284:bool)
              n101 = case shown="Default" "Developer commad" {
                tunnel: [w301 w302 FALSE ("Adquirir") FALSE ("Adquirir")] -> w260
                tunnel: [FALSE ("Adquirir") w302 w303 w305] -> w259
                frame "Adquirir" {
                  w301 = TRUE ("Adquirir")
                  "Adquirir" <- w301
                }
                frame Default {
                  w302 = FALSE ("Adquirir")
                }
                frame "STOP_WHD" {
                  w303 = TRUE ("Adquirir")
                  "Parar la aplicación" <- w303
                }
                frame "Reset_Controlador" {
                  w305 = TRUE ("Adquirir")
                  "Reset del controlador" <- w305
                }
              }
              "Boton Adquirir?" <- w260
              n102 = xnode "Read/Write Control"("FPGA VI Reference In"=w281, "error in"=w280, "Fotocélula"=w260) -> ("FPGA VI Reference Out"=w271:refnum<k20>, "error out"=w270:errorcluster)
              n103 = Select(t="TEST", s=w284, f="Adquisición") -> (s? t:f=w296:string)
              n104 = Select(t="Configuración", s=w259, f=w296) -> (s? t:f=w264:string)
              n105 = Compound Arithmetic op=OR(w260, w284, w259, w274, "Calibration") -> (w261:bool)
              n106 = Select(t="Calibracion", s="Calibration", f=w264) -> (s? t:f=w256:string)
              n107 = Select(t="UPS", s=w253, f=w256) -> (s? t:f=w255:string)
              n108 = Equal?(x="Developer password", y="cafdsadmin") -> (x = y?=w250:bool)
              n109 = property on="Value to compare" class="Arr (strict)"("Visible"=w250) -> ()  [unwired: 2 in, 2 out]
              n110 = property on="mean" class="Arr (strict)"("Visible"=w250) -> ()  [unwired: 2 in, 2 out]
              n111 = property on="median" class="Arr (strict)"("Visible"=w250) -> ()  [unwired: 2 in, 2 out]
              n112 = property on="max" class="Arr (strict)"("Visible"=w250) -> ()  [unwired: 2 in, 2 out]
              n113 = property on="min" class="Arr (strict)"("Visible"=w250) -> ()  [unwired: 2 in, 2 out]
              n114 = property on="Waveform Graph" class="WFGraph (strict)"("Visible"=w250) -> ()  [unwired: 2 in, 2 out]
            }
            n115 = call <vilib>:"Watchdog Clear.vi"("error in (no error)"=w226, "watchdogID in"=w227) -> ("error out"=w225:errorcluster)  [unwired: 5 in]
            n116 = xnode "Read/Write Control"("FPGA VI Reference In"=w220, "error in"=w221) -> ("FPGA VI Reference Out"=w219:refnum<k20>, "error out"=w218:errorcluster, "Direccion 0?"=→"Direccion 0?":bool)
            n117 = Unbundle By Name(w218) -> ("status"=w236:bool)
            n118 = Select(t="TEST", s=w236, f=w237) -> (s? t:f=w232:string)
            n119 = flat-sequence {
              tunnel: [w248] -> w231
              tunnel: w232 -> [w248]
              frame #0 {
                n120 = Get Date/Time In Seconds() -> (seconds since 1Jan1904=w249:timestamp)
                n121 = To Double Precision Float(number=w249) -> (double precision float=→"Tiempo":dbl)
                n122 = local write "Developer commad"("" ("Developer commad")) -> ()
                n123 = local write "Adquirir"(FALSE ("Adquirir")) -> ()
              }
            }
          }
          frame "Adquisición" {
            n124 = local read "Watchdog config"() -> (w323:T1)
            n125 = flat-sequence {
              tunnel: w312 -> [w352]
              tunnel: w311 -> [w351]
              tunnel: [w352] -> w310
              tunnel: [w351] -> w309
              frame #0 {
                n126 = local read "Report"() -> (w348:string)
                n127 = call "Reporting_datetime.vi"() -> ("String"=w347:string)  [unwired: 11 in]
                n128 = Concatenate Strings(w347, "\nSTATUS: ACQUISITION\nTrain is passing\n\n", w348) -> (w350:string)
                n129 = local write "Report"(w350) -> ()
              }
            }
            n130 = call <vilib>:"Watchdog Configure.vi"("error in (no error)"=w322, "expiration actions"=w323, "timeout (1 sec)"=200.0) -> ("error out"=w320:errorcluster, "watchdogID"=w321:u64)  [unwired: 1 in, 2 out]
            n131 = flat-sequence {
              tunnel: w309 -> [w386]
              tunnel: w310 -> [w387]
              tunnel: [w385] -> w337
              tunnel: [w384] -> w336
              tunnel: [w383] -> w335
              tunnel: [w382] -> w334
              tunnel: [w381] -> w333
              tunnel: [w380] -> w332
              tunnel: [w370] -> w325
              tunnel: w321 -> [w369]
              tunnel: w320 -> [w368]
              tunnel: [w369] -> w319
              tunnel: [w368] -> w318
              tunnel: [w402] -> w346
              tunnel: [w419] -> w345
              tunnel: [w418] -> w344
              tunnel: [w417] -> w343
              tunnel: [w410] -> w342
              tunnel: w337 -> [w416]
              tunnel: w336 -> [w415]
              tunnel: w335 -> [w414]
              tunnel: w334 -> [w413]
              tunnel: w333 -> [w412]
              tunnel: w332 -> [w411]
              tunnel: w325 -> [w408]
              tunnel: [w407] -> w324
              tunnel: w319 -> [w406]
              tunnel: w318 -> [w405]
              tunnel: [w403] -> w317
              tunnel: w346 -> [w582]
              tunnel: w345 -> [w579]
              tunnel: w344 -> [w578]
              tunnel: w343 -> [w595]
              tunnel: [w617] -> w329
              tunnel: w342 -> [w619]
              tunnel: [w610] -> w339
              tunnel: [w611] -> w341
              tunnel: [w612] -> w340
              tunnel: w324 -> [w591]
              tunnel: w317 -> [w583]
              tunnel: [w583] -> w315
              tunnel: [w582] -> w314
              frame #0 {
                n132 = local read "Offset_rueda WS 1"() -> (w363:fxp<+/-,24,-4>)
                n133 = local read "Offset_rueda WS 2"() -> (w364:fxp<+/-,24,-4>)
                n134 = local read "Frecuencia de muestreo (Hz)"() -> (w378:dbl)
                n135 = local read "Escaneos de la FIFO por canal"() -> (w367:u32)
                n136 = local read "Canal cero WS1?"() -> (w372:bool)
                n137 = local read "Count(mSec)"() -> (w371:u32)
                n138 = local read "Frecuencia de muestreo y módulo CRIO"() -> (w374:T2)
                n139 = local read "Canal cero WS2"() -> (w362:bool)
                n140 = local read "Digital?"() -> (w373:bool)
                n141 = Get Date/Time In Seconds() -> (seconds since 1Jan1904=→"Inicio pasada":timestamp)
                n142 = local read "Nº de acelerómetros"() -> (w360:i32)
                n143 = local read "Nº inductivos"() -> (w361:i32)
                n144 = xnode "Read/Write Control"("FPGA VI Reference In"=w387, "error in"=w386, "Data Rate"=w374, "Digital?"=w373, "Canal cero WS1?"=w372, "Count(mSec)"=w371, "Offset_WS1"=w363, "Offset_WS2"=w364, "Canal cero WS2?"=w362) -> ("FPGA VI Reference Out"=w377:refnum<k20>, "error out"=w376:errorcluster)
                n145 = local read "RFID LR6 on?"() -> (w365:bool)
                n146 = Add(x=w361, y=w360) -> (x+y=w366:i32)
                n147 = case shown="True" w365 {
                  tunnel: [errorcluster {"status"=FALSE, "code"=0, "source"=""} ("error out") w392] -> w370
                  frame False {
                  }
                  frame True {
                    n148 = local read "RFID_LR6_Error"() -> (w393:errorcluster)
                    n149 = call "LH6HD.vi"("error in (no error)"=w393, "Action"=enum16{"Init", "Start", "Read", "Stop", "Exit"}."Start") -> ("error out"=w392:errorcluster)  [unwired: 8 in, 1 out]
                  }
                }
                n150 = call "DMACalc.vi"("Number of Channels"=w366, "Number of Samples"=w367, "Rate (Hz)"=w378) -> ("Block Size"=w382:u32, "Time to Acquire Block (ms)"=w383:i32, "Host Buffer Size"=w388:u32)  [unwired: 6 in]
                n151 = call "Pathhorafech(SubVI)_varios.vi"("Folder path"=path "c:/Trenes", "Nº de acelerómetros"=w360, "Nº inductivos"=w361) -> ("Acel_Paths"=w356:path[])  [unwired: 1 in, 1 out]
                "Nombre de archivo" <- w356
                n152 = Index Array(array=w356) -> (element=w355:path)  [unwired: 1 in]
                n153 = for {
                  tunnel: w356 -> [w397] mode=indexing
                  tunnel: [w396] -> w381 mode=indexing
                  tunnel: [w395] -> w380
                  n154 = Open/Create/Replace File(file path (use dialog)=w397, operation (0:open)=T4."replace or create", access (0:read/write)=enum16{"read/write", "read-only", "write-only"}."read/write", disable buffering (F)=TRUE) -> (refnum out=w396:refnum<file>, error out=w395:errorcluster)  [unwired: 1 in, 2 out]
                }
                n155 = xnode "Invoke Method"("FPGA VI Reference In"=w377, "error in"=w376, "Requested Depth"=w388) -> ("FPGA VI Reference Out"=w390:refnum<k20>, "error out"=w389:errorcluster)  [unwired: 1 out]
                n156 = local read "Report"() -> (w359:string)
                n157 = Path To String(path=w355) -> (string=w353:string)
                n158 = Concatenate Strings("\nFile created: ", w353, "\n", w359) -> (w358:string)
                n159 = xnode "Invoke Method"("FPGA VI Reference In"=w390, "error in"=w389) -> ("FPGA VI Reference Out"=w385:refnum<k20>, "error out"=w384:errorcluster)
                n160 = local write "Report"(w358) -> ()
              }
              frame #1 {
                n161 = while "Data Acquisition" {
                  tunnel: w416 -> [w470]
                  shift-right: [w494] -> _
                  shift-left: u32 0 ("t") -> [w490]
                  tunnel: w414 -> [w495]
                  tunnel: w413 -> [w493]
                  shift-right: [w496] -> w418
                  shift-left: w415 -> [w487]
                  tunnel: [w491] -> w419
                  tunnel: w412 -> [w474]
                  tunnel: [w475] -> w417
                  shift-right: [w473] -> w410
                  shift-left: w411 -> [w483]
                  stop <- w492 stop-if-true
                  # "Detector de presencia"
                  # "Mide el tiempo de paso del tren y con ello se puede calcular\nla velocidad la unidad"
                  n162 = xnode "Invoke Method"("FPGA VI Reference In"=w470, "error in"=w487, "Number of Elements"=w490, "Timeout (ms)"=0) -> ("FPGA VI Reference Out"=w467:refnum<k20>, "error out"=w472:errorcluster, "Data"=w486:fxp<+/-,24,4>[], "Elements Remaining"=w488:u32)
                  n163 = case "Data Ready" shown="Default" w490 {
                    tunnel: w495 -> [w518 _]
                    tunnel: [w517 u32 0 ("t")] -> w494
                    tunnel: w493 -> [w519 _]
                    tunnel: w488 -> [w516 _]
                    tunnel: w486 -> [_ w541]
                    tunnel: w483 -> [w515 w540]
                    tunnel: [w515 w542] -> w473
                    tunnel: w474 -> [w514 w539]
                    tunnel: [w514 w538] -> w475
                    frame 0 {
                      # "En este caso se compara los elementos que quedan\nen la FIFO del controlador con el tamaño dell bloque\nque aparece en el panel frontal. Si el número de \nelementos en la FIFO es mayor o igual que el tamaño\n del bloque se pasa al siguiente caso y se guardan \nlos datos en un archivo. El reloj que aparece es una\nespera para no consumir recursos."
                      n164 = Greater Or Equal?(x=w516, y=w519) -> (x >= y?=w520:bool)
                      n165 = case shown="False" w520 {
                        tunnel: [u32 0 ("Block Size") w524] -> w517
                        tunnel: [w523 0 ("t")] -> w521
                        tunnel: w518 -> [w523 _]
                        tunnel: w519 -> [_ w524]
                        frame False {
                        }
                        frame True {
                        }
                      }
                      n166 = call "WaitMinTimeBetweenCall.vi"("Minimum ms between calls"=w521) -> ()  [unwired: 2 in]
                    }
                    frame Default {
                      n167 = To Single Precision Float(number=w541) -> (single precision float=w528:sgl[])
                      n168 = Decimate 1D Array(w528) -> (w534:sgl[], w537:sgl[], w536:sgl[], w535:sgl[], w533:sgl[], w532:sgl[], w531:sgl[], w530:sgl[], w529:sgl[], w526:sgl[])
                      n169 = Build Array(w534, w537, w536, w535, w533, w532, w531, w530, w529, w526) -> (w527:sgl[][])
                      n170 = for {
                        tunnel: T5."little-endian" ("byte order (0:big-endian, network order)") -> [w551]
                        shift-right: [w545] -> w542
                        shift-left: w540 -> [w546]
                        tunnel: w527 -> [w549] mode=indexing
                        tunnel: w539 -> [w548] mode=indexing
                        tunnel: [w547] -> w538 mode=indexing
                        n171 = Write to Binary File(file (use dialog)=w548, data=w549, error in=w546, 5:FALSE ("prepend array or string size? (T)"), 9:w551) -> (refnum out=w547:refnum<file>, error out=w545:errorcluster)  [unwired: 2 out]
                      }
                    }
                  }
                  n172 = xnode "Read/Write Control"("FPGA VI Reference In"=w467, "error in"=w472) -> ("FPGA VI Reference Out"=w485:refnum<k20>, "error out"=w484:errorcluster, "Parar"=w463:bool, "Nº Ruedas 1"=→"Nº Ruedas 1":i32, "NºRuedas 2"=→"NºRuedas 2":i32)
                  "Parar" <- w463
                  n173 = case shown="False" w463 {
                    tunnel: [w501 w509] -> w464
                    tunnel: [w502 0.0] -> w478
                    frame False {
                      n174 = local read "Inicio pasada"() -> (w505:timestamp)
                      n175 = Get Date/Time In Seconds() -> (seconds since 1Jan1904=w504:timestamp)
                      n176 = local read "Tiempo de adquisicion"() -> (w497:dbl)
                      n177 = To Double Precision Float(number=w504) -> (double precision float=w503:dbl)
                      n178 = To Double Precision Float(number=w505) -> (double precision float=w506:dbl)
                      n179 = Subtract(x=w503, y=w506) -> (x-y=w502:dbl)
                      "Tiempo de paso (s)" <- w502
                      n180 = local write "Tiempo"(w503) -> ()
                      n181 = local read "Boton Adquirir?"() -> (w498:bool)
                      n182 = Greater?(x=w502, y=w497) -> (0:w500:bool)
                      n183 = Select(t=w500, s=w498, f=FALSE) -> (s? t:f=w501:bool)
                    }
                    frame True {
                      n184 = local read "Tiempo"() -> (w513:dbl)
                      n185 = local read "Tiempo extra al detector de paso (s)"() -> (w508:dbl)
                      n186 = Get Date/Time In Seconds() -> (seconds since 1Jan1904=w510:timestamp)
                      n187 = To Double Precision Float(number=w510) -> (double precision float=w511:dbl)
                      n188 = Subtract(x=w511, y=w513) -> (x-y=w512:dbl)
                      n189 = Greater?(x=w512, y=w508) -> (0:w509:bool)
                    }
                  }
                  "Fin" <- w464
                  n190 = local read "Timeout ruedas"() -> (w462:dbl)
                  n191 = xnode ("CheckLate")("FPGA VI Reference In"=w485, "error in"=w484) -> ("FPGA VI Reference Out"=w469:refnum<k20>, "error out"=w480:errorcluster, "Buffer Underflow"=→"Buffer Underflow":bool, "Buffer Overflow"=w471:bool)
                  "Buffer Overflow" <- w471
                  n192 = Greater?(x=w478, y=w462) -> (0:w476:bool)
                  "Timeout ruedas" <- w476
                  n193 = call "ErrorOverFlow.vi"("Buffer Overflow"=w471) -> ("error out"=w479:errorcluster)
                  n194 = Merge Errors(w480, w479) -> (w468:errorcluster)
                  n195 = Unbundle By Name(w473) -> ("status"=w477:bool)
                  n196 = Unbundle By Name(w468) -> ("status"=w482:bool)
                  n197 = Compound Arithmetic op=OR(w482, w464, w476, w477) -> (w492:bool)
                  "result" <- w492
                  n198 = case "Flush" shown="True" w492 {
                    tunnel: [w552 w557] -> w496
                    tunnel: [w553 w556] -> w491
                    tunnel: w469 -> [w553 w555]
                    tunnel: w468 -> [w552 w554]
                    frame False {
                    }
                    frame True {
                      n199 = xnode "Invoke Method"("FPGA VI Reference In"=w555, "error in"=w554) -> ("FPGA VI Reference Out"=w556:refnum<k20>, "error out"=w557:errorcluster)
                    }
                  }
                  "Block Size" <- w493
                  "Time to Acquire Block (ms)" <- w495
                }
                n200 = call <vilib>:"Watchdog Whack.vi"("error in (no error)"=w405, "reset watchdog after expire? (F)"=TRUE, "watchdogID in"=w406) -> ("error out"=w402:errorcluster, "watchdogID out"=w403:u64)  [unwired: 2 in, 1 out]
                n201 = local read "RFID LR6 on?"() -> (w401:bool)
                n202 = case shown="True" w401 {
                  tunnel: w408 -> [w420 w426]
                  tunnel: [w420 w425] -> w407
                  frame False {
                  }
                  frame True {
                    n203 = while {
                      shift-right: [w433] -> w425
                      shift-left: w426 -> [w434]
                      shift-right: [w432] -> w423
                      shift-left: string[] [] -> [w431]
                      shift-right: [w427] -> w421
                      shift-left: i32[] [] -> [w428]
                      i -> [w429]
                      stop <- w430 stop-if-true
                      n204 = case shown="No Error" w434 {
                        selector: w434 -> [w445 _]
                        tunnel: [w444 w460] -> w433
                        tunnel: [w440 string[] []] -> w432
                        tunnel: w431 -> [w439 _]
                        tunnel: w429 -> [w438 _]
                        tunnel: w428 -> [w437 _]
                        tunnel: [w436 i32[] []] -> w427
                        frame No Error {
                          n205 = call "LH6HD.vi"("error in (no error)"=w445, "Action"=enum16{"Init", "Start", "Read", "Stop", "Exit"}."Read") -> ("error out"=w444:errorcluster, "Tag"=w441:string)  [unwired: 8 in]
                          n206 = Not Equal?(x="", y=w441) -> (x != y?=w442:bool)
                          n207 = case shown="False" w442 {
                            tunnel: w441 -> [_ w454]
                            tunnel: [w448 w453] -> w440
                            tunnel: w439 -> [w448 w452]
                            tunnel: w438 -> [_ w449]
                            tunnel: w437 -> [w447 w451]
                            tunnel: [w447 w450] -> w436
                            frame False {
                            }
                            frame True {
                              n208 = Build Array (concatenate)(w452, w454) -> (w453:string[])
                              n209 = Build Array (concatenate)(w451, w449) -> (w450:i32[])
                            }
                          }
                        }
                        frame Error {
                          n210 = local read "LR6 IP address"() -> (w457:string)
                          n211 = local read "DeviceAddress"() -> (w455:u8)
                          n212 = local read "Port LR6"() -> (w458:u16)
                          n213 = call "LH6HD.vi"("DeviceAddress"=w455, "Reader Port"=w458, "IP Address"=w457, "Action"=enum16{"Init", "Start", "Read", "Stop", "Exit"}."Init") -> ("error out"=w460:errorcluster)  [unwired: 6 in, 1 out]
                        }
                      }
                      n214 = Wait Until Next ms Multiple(millisecond multiple=u32 500) -> ()  [unwired: 1 out]
                      n215 = local read "result"() -> (w430:bool)
                      "it-LR6" <- w429
                    }
                    "TAGs LR6" <- w423
                    "it-read-LR6" <- w421
                  }
                }
              }
              frame #2 {
                # "ORGANIZAR\nTAGS AQUÍ"
                n216 = local read "RFID LR6 on?"() -> (w580:bool)
                n217 = local read "RFID NEM on?"() -> (w581:bool)
                n218 = Array Size(array=w595) -> (size(s)=w593:i32)
                n219 = local read "AURA wheel test"() -> (w561:bool)
                n220 = Decrement(x=w593) -> (x-1=w594:i32)
                n221 = case shown="True" w580 {
                  tunnel: w591 -> [w625 w631]
                  tunnel: [w625 w626] -> w590
                  frame False {
                  }
                  frame True {
                    n222 = call "LH6HD.vi"("error in (no error)"=w631, "Action"=enum16{"Init", "Start", "Read", "Stop", "Exit"}."Stop") -> ("error out"=w626:errorcluster)  [unwired: 8 in, 1 out]
                    n223 = call "Reporting_error.vi"("error out 2"=w626, "Concept"="Active RFID") -> ("Reporting"=w628:string)  [unwired: 1 in]
                    n224 = local read "Report"() -> (w629:string)
                    n225 = Concatenate Strings(w628, w629) -> (w627:string)
                    n226 = local write "Report"(w627) -> ()
                  }
                }
                n227 = case shown="True" w581 {
                  tunnel: [string[] [] ("TagArray") w638] -> w559
                  tunnel: [cluster{"TagCode":string, "FirstSeemUs":u64}[] [] ("TagData out") w637] -> w558
                  frame False {
                  }
                  frame True {
                    n228 = call "IF2_TagBuffer.vi"("Action"=enum16{"Init", "WriteTagData", "ReadTagData"}."ReadTagData") -> ("error out"=w636:errorcluster, "TagData out"=w637:cluster{"TagCode":string, "FirstSeemUs":u64}[])  [unwired: 9 in]
                    n229 = local read "connection ID"() -> (w635:refnum<k5>)
                    n230 = call "RFID_TAGS_Sort.vi"("TagData in"=w637) -> ("TagString"=w639:string, "TagArray"=w638:string[])  [unwired: 9 in]
                    n231 = call "IF2_Clear_buffer.vi"("error in (no error)"=w636, "TCP Network Connection in"=w635) -> ()  [unwired: 8 in, 2 out]
                    n232 = call "Reporting_error.vi"("error out 2"=w636, "Concept explanation"=w639, "Concept"="Passive RFID") -> ("Reporting"=w642:string)
                    n233 = local read "Report"() -> (w643:string)
                    n234 = Concatenate Strings(w642, w643) -> (w641:string)
                    n235 = local write "Report"(w641) -> ()
                  }
                }
                "TAGs HEX" <- w559
                n236 = Index Array(array=w595, index=w594) -> (element=w603:refnum<file>)
                n237 = local write "result"(FALSE ("result")) -> ()
                n238 = xnode "Read/Write Control"("FPGA VI Reference In"=w579, "error in"=w578) -> ("FPGA VI Reference Out"=w616:refnum<k20>, "error out"=w576:errorcluster, "Chassis Temperature"=w624:i16)
                n239 = local read "TAGs LR6"() -> (w563:string[])
                n240 = Select(t=string[] ["A0000000000000000TESTNEM7", "A0000000000000000TESTNEM8"], s=w561, f=w563) -> (s? t:f=w560:string[])
                n241 = Divide(x=w624, y=4.0) -> (x/y=w572:dbl)
                "Temperatura (ºC)" <- w572
                n242 = local read "Tiempo de paso (s)"() -> (w614:dbl)
                n243 = for {
                  tunnel: w560 -> [w647] mode=indexing
                  tunnel: [w645] -> w584 mode=indexing
                  n244 = Search and Replace String(input string=w647, search string="00") -> (result string=w645:string)  [unwired: 6 in, 3 out]
                }
                n245 = local write "RFID_LR6_Error"(w590) -> ()
                n246 = Index Array(array=w559) -> (element=w589:string)  [unwired: 1 in]
                n247 = local read "Nº Ruedas 1"() -> (w570:i32)
                n248 = local read "NºRuedas 2"() -> (w574:i32)
                n249 = Not Equal?(x=w589, y="" ("delimiter (\\t)")) -> (x != y?=w587:bool)
                "Plataformas?" <- w587
                n250 = Multiply(x=w614, y=1000.0) -> (x*y=w571:dbl)
                n251 = case shown="True" w587 {
                  tunnel: w584 -> [w648 w654]
                  tunnel: [w648 w653] -> w573
                  tunnel: w559 -> [_ _]
                  tunnel: w558 -> [_ w649]
                  frame False {
                  }
                  frame True {
                    n252 = local read "Tiempo de paso (s)"() -> (w651:dbl)
                    n253 = local read "Tabla_flota"() -> (w650:string[][])
                    n254 = local read "Inicio pasada"() -> (w652:timestamp)
                    n255 = call "Union_TAGs_RFIDs.vi"("TAGs LR6"=w654) -> ()  [unwired: 1 in, 1 out]
                    n256 = call "TagNormalizaction.vi"("Inicio pasada"=w652, "Tiempo de paso (s)"=w651, "TagData in"=w649, "Tabla_flota"=w650) -> ("Normalized Tags"=w653:string[])  [unwired: 7 in]
                  }
                }
                "TAGs" <- w573
                n257 = Build Array(w572, w571, w570, w574) -> (w575:dbl[])
                n258 = Build Array(w572, w571, w570) -> (w569:dbl[])
                n259 = local read "Direccion 0?"() -> (w568:bool)
                n260 = local read "Nombre de archivo"() -> (w602:path[])
                n261 = Bundle("error out"=w576, w575, "Normalized Tags"=w573, "Direccion 0?"=w568) -> (w567:T10)  [unwired: 1 in]
                n262 = for {
                  shift-right: [w660] -> w608
                  shift-left: string[] [] -> [w659]
                  tunnel: w573 -> [w658] mode=indexing
                  n263 = Insert Into Array(array=w659, new element=w658) -> (w660:string[])  [unwired: 1 in]
                }
                n264 = xnode "Read/Write Control"("FPGA VI Reference In"=w616, "error in"=w576, "Stop"=TRUE ("stop")) -> ("FPGA VI Reference Out"=w605:refnum<k20>, "error out"=w604:errorcluster)
                n265 = call "Reporting_acqu.vi"("output cluster"=w567, "address repoting"=path "C:/Reporting/Reporting_adqu.txt" ("file (use dialog)")) -> ("Reporting"=w564:string)  [unwired: 1 in]
                n266 = Delete From Array(array=w602) -> (deleted portion=w601:path)  [unwired: 2 in, 1 out]
                n267 = local read "Report"() -> (w565:string)
                n268 = To Single Precision Float(number=w569) -> (single precision float=w622:sgl[])
                n269 = Path To String(path=w601) -> (string=w607:string)
                n270 = Concatenate Strings(w564, w565) -> (w566:string)
                n271 = Write to Binary File(file (use dialog)=w603, data=w622, error in=w619, 5:FALSE ("prepend array or string size? (T)"), 9:T5."little-endian" ("byte order (0:big-endian, network order)")) -> (error out=w600:errorcluster)  [unwired: 3 out]
                n272 = xnode "Invoke Method"("FPGA VI Reference In"=w605, "error in"=w604) -> ("FPGA VI Reference Out"=w612:refnum<k20>, "error out"=w611:errorcluster)
                n273 = local read "Timeout ruedas"() -> (w615:bool)
                n274 = local write "Report"(w566) -> ()
                n275 = Build Array (concatenate)(w607, w608) -> (w585:string[])
                n276 = local read "TAGS leidos"() -> (w596:path)
                n277 = for {
                  shift-right: [w657] -> w610
                  shift-left: w600 -> [w656]
                  tunnel: w595 -> [w655] mode=indexing
                  n278 = Close File(refnum=w655, error in=w656) -> (error out=w657:errorcluster)  [unwired: 1 out]
                }
                n279 = call-poly <vilib>:"Write Delimited Spreadsheet.vi"("file path (dialog if empty)"=w596, "1D data"=w585, "append to file? (F)"=TRUE ("transpose? (no:F)"), "transpose? (F)"=TRUE ("append to file? (new file:F)"), "delimiter (\\t)"=";" ("delimiter (\\t)")) -> ()  [unwired: 9 in, 2 out]
                n280 = Select(t="TEST", s=w615, f="Procesado") -> (s? t:f=w617:string)
              }
            }
            n281 = call <vilib>:"Watchdog Clear.vi"("error in (no error)"=w314, "watchdogID in"=w315) -> ("error out"=w316:errorcluster)  [unwired: 5 in]
            n282 = Unbundle By Name(w341) -> ("status"=w330:bool)
            n283 = Unbundle By Name(w339) -> ("status"=w331:bool)
            n284 = Merge Errors(w339, w316) -> (w338:errorcluster)
            n285 = Compound Arithmetic op=OR(w330, w331) -> (w328:bool)
            n286 = Select(t="TEST", s=w328, f=w329) -> (s? t:f=w326:string)
          }
          frame "Procesado" {
            n287 = local read "Watchdog config"() -> (w672:T1)
            n288 = flat-sequence {
              tunnel: w666 -> [w685]
              tunnel: [w685] -> w665
              tunnel: w664 -> [w681]
              tunnel: [w681] -> w663
              frame #0 {
                n289 = local read "Report"() -> (w682:string)
                n290 = call "Reporting_datetime.vi"() -> ("String"=w680:string)  [unwired: 11 in]
                n291 = Concatenate Strings(w680, "\nSTATUS: PROCESSING\nProcessing the measurement\n\n", w682) -> (w684:string)
                n292 = local write "Report"(w684) -> ()
              }
            }
            n293 = call <vilib>:"Watchdog Configure.vi"("error in (no error)"=w675, "expiration actions"=w672, "timeout (1 sec)"=300.0) -> ("error out"=w674:errorcluster, "watchdogID"=w671:u64)  [unwired: 1 in, 2 out]
            n294 = flat-sequence {
              tunnel: w674 -> [w692]
              tunnel: w671 -> [w688]
              tunnel: [w687] -> w670
              tunnel: [w686] -> w669
              tunnel: [w903] -> w668
              tunnel: w670 -> [w903]
              tunnel: [w902] -> w667
              tunnel: w669 -> [w902]
              frame #0 {
                n295 = flat-sequence {
                  tunnel: [w764] -> w694
                  tunnel: [w750] -> w693
                  tunnel: w692 -> [w731]
                  tunnel: [w713] -> w689
                  tunnel: [w752] -> w691
                  tunnel: [w704] -> w690
                  tunnel: w688 -> [w732]
                  tunnel: [w729] -> w687
                  tunnel: [w728] -> w686
                  frame #0 {
                    n296 = local read "AURA wheel test"() -> (w702:bool)
                    n297 = case shown="False" w702 {
                      tunnel: [w767 w768] -> w701
                      tunnel: [w766 path[] [path "c:/Trenes_prueba/A_0_TEST.bin", path "c:/Trenes_prueba/A_1_TEST.bin", path "c:/Trenes_prueba/A_2_TEST.bin", path "c:/Trenes_prueba/A_3_TEST.bin", path "c:/Trenes_prueba/A_4_TEST.bin", path "c:/Trenes_prueba/A_5_TEST.bin", path "c:/Trenes_prueba/A_6_TEST.bin", path "c:/Trenes_prueba/A_7_TEST.bin", path "c:/Trenes_prueba/I_0_TEST.bin", path "c:/Trenes_prueba/I_1_TEST.bin"]] -> w700
                      frame False {
                        n298 = local read "Nombre de archivo"() -> (w766:path[])
                        n299 = local read "TAGs"() -> (w767:string[])
                      }
                      frame True {
                        w768 = string[] ["A0000000000000000TESTNEM7", "A0000000000000000TESTNEM8"]
                        n300 = local write "TAGs LR6"(w768) -> ()
                      }
                    }
                    n301 = local read "Tabla_flota"() -> (w749:string[][])
                    n302 = call <vilib>:"Watchdog Whack.vi"("error in (no error)"=w731, "reset watchdog after expire? (F)"=TRUE, "watchdogID in"=w732) -> ("error out"=w728:errorcluster, "watchdogID out"=w729:u64)  [unwired: 2 in, 1 out]
                    n303 = local read "Puntos medios de las ventanas"() -> (w751:dbl[][])
                    n304 = call "Series_ejes_flota.vi"("Tabla_flota"=w749, "Tags"=w701) -> ("Nº Ejes"=w726:i32[], "Series del convoy"=w743:string[])  [unwired: 2 in, 1 out]
                    "Nº Ejes" <- w726
                    n305 = Array Size(array=w700) -> (size(s)=w758:i32)
                    n306 = Add Array Elements(numeric array=w726) -> (sum=w712:i32)
                    "Ejes_convoy" <- w712
                    n307 = Subtract(x=w758, y=2 ("length")) -> (x-y=w760:i32)
                    n308 = Array Size(array=w743) -> (size(s)=→"Nº UTs":i32)
                    n309 = local read "Series_flota"() -> (w748:string[])
                    n310 = Delete From Array(array=w700, length=2, index=w760) -> (deleted portion=w733:path[], array with subset deleted=w752:path[])
                    n311 = Index Array(array=w733) -> (element #2=w727:path)  [unwired: 2 in, 1 out]
                    n312 = call "Distancias_ejes_convoy.vi"("Series_flota1"=w743, "Ejes_UT"=w726, "Puntos medios de las ventanas"=w751, "Series_flota"=w748) -> ("Distancias_entre_ejes_convoy"=w750:dbl[])  [unwired: 1 in]
                    n313 = Read from Binary File(5:sgl 0.0, 9:T5."little-endian" ("byte order (0:big-endian, network order)"), 10:-1 ("count (1)"), 11:w727) -> (0:w756:errorcluster, 2:w735:sgl[], 3:w757:refnum<file>)  [unwired: 1 in, 2 out]
                    n314 = local read "Frecuencia de muestreo (Hz)"() -> (w717:dbl)
                    n315 = local read "Offset_rueda WS 2"() -> (w718:fxp<+/-,24,-4>)
                    n316 = local read "it-LR6"() -> (w738:i32)
                    n317 = local read "it-read-LR6"() -> (w739:i32[])
                    n318 = local read "Plataformas?"() -> (w737:bool)
                    n319 = local read "TAGs"() -> (w741:string[])
                    n320 = local read "TAGs LR6"() -> (w740:string[])
                    n321 = Close File(refnum=w757, error in=w756) -> (error out=w696:errorcluster)  [unwired: 1 out]
                    n322 = Array Size(array=w735) -> (size(s)=w747:i32)
                    n323 = Subtract(x=w747, y=3 ("length")) -> (x-y=w745:i32)
                    n324 = Delete From Array(array=w735, length=3, index=w745) -> (array with subset deleted=w724:sgl[])  [unwired: 1 out]
                    n325 = call "TAGs_AURAwheel_TAGM_NEM.vi"("Nº Ejes"=w726, "TAGs"=w741, "Ejes_convoy"=w712, "it-LR6"=w738, "TAGs LR6"=w740, "it-read-LR6"=w739, "Plataformas?"=w737) -> ("TAGS_AURA"=→"TAGs_AURAwheel":string[][])  [unwired: 1 in]
                    n326 = call "Analogico_digital.vi"("Array"=w724, "Offset WS"=w718, "Frecuencia muestreo"=w717) -> ("array w/ subset deleted"=w719:sgl[], "Tiempo\npaso"=w716:dbl)  [unwired: 6 in]
                    n327 = call "Puntos medio de pulso.vi"("DI Inductivo"=w719) -> ("Puntos"=w764:sgl[], "Número de ejes"=w706:i32)  [unwired: 1 in]
                    "Número de ejes detectados" <- w706
                    n328 = disable-structure shown="Enabled" {
                      disable-tunnel: w724 -> [w776 w779]
                      disable-tunnel: [FALSE ("element") TRUE ("element")] -> w721
                      disable-tunnel: [w770 w778] -> w720
                      frame Disabled {
                        n329 = Equal?(x=w776, y=0.0) -> (x = y?=w773:bool[])
                        n330 = Equal?(x=w776, y=1.0) -> (x = y?=w774:bool[])
                        n331 = Or(x=w773, y=w774) -> (x .or. y?=w770:bool[])
                      }
                      frame Enabled {
                        n332 = Greater?(x=w779, y=0.1) -> (0:w778:bool[])
                      }
                    }
                    n333 = Decrement(x=w706) -> (x-1=w763:i32)
                    n334 = call "Reporting_error.vi"("error out 2"=w696, "Concept"="Measurement reading") -> ("Reporting"=w698:string)  [unwired: 1 in]
                    n335 = Get Volume Info(11:path "c:/" ("path")) -> (1:w707:i64)  [unwired: 1 in, 5 out]
                    "Disco Duro Disponible (bytes)" <- w707
                    n336 = local read "Report"() -> (w699:string)
                    n337 = call "Calculo_Velocidad.vi"("Tiempo de paso (s)"=w716, "Ejes"=w763, "Puntos iniciales de las ventanas"=w750) -> ("V (m/s)"=→"V (m/s)":dbl, "Longitud de la unidad"=→"Longitud de la unidad":dbl)
                    n338 = Concatenate Strings(w698, w699) -> (w697:string)
                    n339 = Equal?(x=w712, y=w706) -> (x = y?=w704:bool)
                    n340 = Not Equal?(x=w706, y=0) -> (x != y?=w703:bool)
                    n341 = Search 1D Array(1D array=w720, element=w721) -> (index of element=w722:i32)  [unwired: 1 in]
                    n342 = local write "Report"(w697) -> ()
                    n343 = Build Array(w712, w706, w707) -> (w711:i64[])
                    n344 = Equal?(x=w722, y=-1) -> (x = y?=w725:bool)
                    n345 = Compound Arithmetic op=AND(w704, w703, w725) -> (w713:bool)
                    "Archivo\nvalido?" <- w713
                    n346 = Bundle(w711, w713) -> (w709:cluster{i64[], bool})  [unwired: 1 in]
                    n347 = call "Reporting_proc.vi"("output cluster 2"=w709, "address repoting"=path "C:/Reporting/Reporting_proc.txt" ("file (use dialog)")) -> ("Reporting"=w708:string)  [unwired: 1 in]
                    n348 = local read "Report"() -> (w714:string)
                    n349 = Concatenate Strings(w708, w714) -> (w715:string)
                    n350 = local write "Report"(w715) -> ()
                  }
                }
                n351 = case shown="True" w689 {
                  tunnel: w694 -> [_ w814]
                  tunnel: w693 -> [_ w812]
                  tunnel: w691 -> [_ w813]
                  tunnel: w690 -> [w781 _]
                  frame False {
                    n352 = local read "Nombre de archivo"() -> (w782:path[])
                    n353 = for {
                      tunnel: w782 -> [w784] mode=indexing
                      tunnel: w781 -> [w783]
                      n354 = flat-sequence {
                        tunnel: w784 -> [w794]
                        tunnel: [w794] -> w787
                        tunnel: [w793] -> w786
                        tunnel: w783 -> [w792]
                        tunnel: w787 -> [w801]
                        tunnel: [w800] -> w785
                        tunnel: w786 -> [w800]
                        tunnel: w785 -> [w803]
                        frame #0 {
                          w793 = path "c:/Est_Adq.csv" ("file path (use dialog)")
                          n355 = Path To String(path=w794) -> (string=w795:string)
                          n356 = Select(t="Nº Ejes detectados WS diferente a Nº Ejes TAGs" ("delimiter (\\t)"), s=w792, f="La señal del inductivo no es digital" ("delimiter (\\t)")) -> (s? t:f=w789:string)
                          n357 = Build Array(w795, w789) -> (w788:string[])
                          n358 = call-poly <vilib>:"Write Delimited Spreadsheet.vi"("file path (dialog if empty)"=w793, "1D data"=w788, "append to file? (F)"=FALSE ("transpose? (no:F)"), "transpose? (F)"=TRUE ("append to file? (new file:F)"), "delimiter (\\t)"=";" ("delimiter (\\t)")) -> ()  [unwired: 9 in, 2 out]
                        }
                        frame #1 {
                          n359 = local read "Borrar archivos\nadquisicion con error"() -> (w799:bool)
                          n360 = case shown="True" w799 {
                            tunnel: w801 -> [_ w802]
                            frame False {
                            }
                            frame True {
                              n361 = Delete(path (use dialog)=w802) -> ()  [unwired: 1 in, 6 out]
                            }
                          }
                        }
                        frame #2 {
                          n362 = File/Directory Info(path=w803) -> (size=w806:i64)  [unwired: 1 in, 6 out]
                          n363 = Greater?(x=w806, y=i64 1000000) -> (0:w804:bool)
                          n364 = case shown="True" w804 {
                            tunnel: w803 -> [_ w807]
                            frame False {
                            }
                            frame True {
                              n365 = Delete(path (use dialog)=w807) -> ()  [unwired: 4 in, 3 out]
                            }
                          }
                        }
                      }
                    }
                  }
                  frame True {
                    n366 = flat-sequence {
                      tunnel: w814 -> [w891]
                      tunnel: w813 -> [w888]
                      tunnel: w812 -> [w892]
                      tunnel: [w875] -> w811
                      frame #0 {
                        # "SALIDA \n\nMáximos por rueda inductivo"
                        # "8 acelerómetros"
                        # "Velocidad"
                        n367 = local read "Frecuencia de muestreo (Hz)"() -> (w890:dbl)
                        n368 = local read "Distancia de acelerómetros"() -> (w880:dbl[])
                        n369 = local read "Parámetros acelerómetros"() -> (w887:dbl[])
                        n370 = local read "Número de ejes detectados"() -> (w886:i32)
                        n371 = local read "Distancias generales"() -> (w885:dbl[])
                        n372 = local read "dt RMS"() -> (w889:dbl)
                        n373 = local read "Direccion 0?"() -> (w877:bool)
                        n374 = Index Array(array=w885, index=1) -> (element=w883:dbl)
                        n375 = Select(t=0.0, s=w877, f=w883) -> (s? t:f=w881:dbl)
                        n376 = Subtract(x=w881, y=w880) -> (x-y=w879:dbl[])
                        n377 = Absolute Value(x=w879) -> (abs(x)=w878:dbl[])
                        n378 = call "Procesado_aRMS_BIdirecc.vi"("Paths_canales_aRMS"=w888, "Ejes Procesados"=w886, "Distancias\nacelerometros"=w878, "Distancias generales (m)"=w885, "Distancias centrales de las ruedas\n               configuración (m)"=w892, "Frecuencia de muestreo"=w890, "Parámetros acelerómetros"=w887, "dt RMS 2"=w889, "Puntos"=w891) -> ("Max RMS Ruedas"=w876:dbl[][])  [unwired: 2 in]
                        n379 = Transpose 2D Array(2D array=w876) -> (transposed array=w875:dbl[][])
                        "Max RMS Ruedas" <- w875
                        n380 = call "Reporting_proc_RMS.vi"("Max RMS Ruedas"=w875) -> ("String"=w873:string)
                        n381 = local read "Report"() -> (w874:string)
                        n382 = Concatenate Strings(w873, w874) -> (w872:string)
                        n383 = local write "Report"(w872) -> ()
                      }
                    }
                    n384 = local read "Use Aura?"() -> (w810:bool)
                    n385 = local read "TAGs_AURAwheel"() -> (w809:string[][])
                    n386 = local read "Nº Ejes"() -> (w808:i32[])
                    n387 = for {
                      tunnel: w810 -> [w818]
                      tunnel: w809 -> [w817] mode=indexing
                      shift-right: [w816] -> _
                      shift-left: w811 -> [w819]
                      tunnel: w808 -> [w815] mode=indexing
                      # "dev.api.aurawheel.com"
                      n388 = case shown="True" w818 {
                        tunnel: w819 -> [w820 w839]
                        tunnel: w817 -> [_ w840]
                        tunnel: [w820 w838] -> w816
                        tunnel: w815 -> [_ w836]
                        frame False {
                        }
                        frame True {
                          w824 = "\n"
                          w847 = cluster{"status":string} {"status"=""}
                          n389 = local read "Parametros AuraWheel"() -> (w871:string[])
                          n390 = Delete From Array(array=w839, length=w836, index (row)=0) -> (deleted portion=w835:dbl[][], array with subset deleted=w838:dbl[][])  [unwired: 1 in]
                          n391 = Get Date/Time In Seconds() -> (seconds since 1Jan1904=w868:timestamp)
                          n392 = Format Date/Time String(time format string (%c)="%H:%M:%S%3u", seconds (now)=w868) -> (date/time string=w866:string)  [unwired: 1 in]
                          n393 = Get Date/Time In Seconds() -> (seconds since 1Jan1904=w843:timestamp)
                          n394 = Scan From String(format string="%d:%d:%f", input string=w866) -> (output 1=w863:i32, output 2=w862:i32, output 3=w860:dbl)  [unwired: 5 in, 3 out]
                          n395 = local read "V (m/s)"() -> (w831:dbl)
                          n396 = local read "Temperatura (ºC)"() -> (w841:dbl)
                          n397 = Multiply(x=w831, y=3.6) -> (x*y=w829:dbl)
                          n398 = Multiply(x=w860, y=1000.0) -> (x*y=w856:dbl)
                          n399 = call "Time_to_ms.vi"("seconds since 1Jan1904"=w843) -> ("Numeric"=w842:dbl)  [unwired: 1 in]
                          n400 = Multiply(x=w862, y=60000) -> (x*y=w857:i32)
                          n401 = Multiply(x=3600000, y=w863) -> (x*y=w858:i32)
                          n402 = Index Array(array=w871) -> (element #1=w834:string, element #2=w833:string, element #3=w832:string)  [unwired: 3 in]
                          n403 = call "aw_WRDCluster_8acel.vi"("Array TAGs"=w840, "Max RMS Ruedas"=w835, "TimeStamp"=w842, "p_sp"=w829, "p_tp"=w841) -> ("JSON cluster"=w869:T11)  [unwired: 1 in]
                          n404 = Compound Arithmetic op=ADD(w858, w857, w856) -> (w855:dbl)
                          n405 = To Variant(anything=w869) -> (Variant=w852:variant)
                          n406 = To Unsigned Long Integer(number=w855) -> (unsigned 32bit integer=w854:u32)
                          n407 = call "gjson_Create.vi"("JSON Object in"=w852) -> ("error out"=w850:errorcluster, "JSON String Out"=w851:string)  [unwired: 9 in]
                          n408 = Number To Decimal String(number=w854) -> (decimal integer string=w853:string)  [unwired: 1 in]
                          n409 = To Variant(anything=w847) -> (Variant=w846:variant)
                          n410 = call "aw_SendData.vi"("pwd"=w834, "x-nem-datetime"=w853, "User"=w833, "error in"=w850, "JSON Object"=w851, "URL"=w832) -> ("error out"=w848:errorcluster, "Response JSON"=w849:string, "Response headers"=w825:string)  [unwired: 3 in]
                          "Response headers" <- w825
                          n411 = call "gjson_Parse.vi"("error in"=w848, "JSON String In"=w849, "JSON Cluster"=w846) -> ("error out"=w844:errorcluster, "JSON Cluster Out"=w845:variant)  [unwired: 7 in]
                          n412 = Variant To Data(error in=w844, type=w847, Variant=w845) -> (data=→"data":cluster{"status":string}, error out=w826:errorcluster)
                          "error AURA" <- w826
                          n413 = local read "Report"() -> (w822:string)
                          n414 = call "Reporting_error.vi"("error out 2"=w826, "Concept"="A.U.R.A. Wheel Connection") -> ("Reporting"=w827:string)  [unwired: 1 in]
                          n415 = Concatenate Strings(w827, w824, w824, w825, w824) -> (w823:string)
                          "Report_AURA" <- w823
                          n416 = Concatenate Strings(w823, w822) -> (w821:string)
                          n417 = local write "Report"(w821) -> ()
                        }
                      }
                    }
                  }
                }
              }
              frame #1 {
                n418 = local read "Archivo\nvalido?"() -> (w899:bool)
                n419 = local read "Bytes libre despues de borrar"() -> (w900:u32)
                n420 = local read "Report_AURA"() -> (w896:string)
                n421 = local read "Max archivos"() -> (w897:u32)
                n422 = local read "Path LOG"() -> (w898:path)
                n423 = local read "LOG.txt"() -> (w893:path)
                n424 = local read "Report"() -> (w895:string)
                n425 = local read "Bytes min libre"() -> (w901:u32)
                n426 = local read "TAGS leidos"() -> (w904:path)
                n427 = File/Directory Info(path=w904) -> (size=w907:i64)  [unwired: 1 in, 6 out]
                n428 = case shown="True" w899 {
                  frame False {
                  }
                  frame True {
                    n429 = local read "Nombre de archivo"() -> (w909:path[])
                    n430 = call "Comprimir_a_1_archivo.vi"("Acel_paths"=w909) -> ("path_Pasada"=→"created path":path)
                  }
                }
                n431 = Greater?(x=w907, y=i64 1000000) -> (0:w905:bool)
                n432 = case shown="True" w905 {
                  tunnel: w904 -> [_ w910]
                  frame False {
                  }
                  frame True {
                    n433 = Delete(path (use dialog)=w910) -> ()  [unwired: 4 in, 3 out]
                  }
                }
                n434 = call "BORRADO_MEJORADO_Gonzalo.vi"("Bytes LIBRE OK"=w900, "Bytes Minimo de Memoria libre"=w901) -> ()  [unwired: 10 in]
                n435 = call "Saving_LOG.vi"("Path"=w893, "Report"=w895, "Report AURA"=w896, "Path Carpeta"=w898, "Nº Archivos Max"=w897) -> ("Report"=w894:string)  [unwired: 9 in, 1 out]
                n436 = local write "Report"(w894) -> ()
              }
            }
            n437 = call <vilib>:"Watchdog Clear.vi"("error in (no error)"=w667, "watchdogID in"=w668) -> ("error out"=w661:errorcluster)  [unwired: 5 in]
            n438 = Merge Errors(w663, w661) -> (w679:errorcluster)
            n439 = Unbundle By Name(w679) -> ("status"=w677:bool)
            n440 = Select(t="TEST", s=w677, f="Espera") -> (s? t:f=w676:string)
          }
          frame "TEST" {
            n441 = flat-sequence {
              tunnel: [w926] -> w913
              tunnel: w915 -> [w926]
              frame #0 {
                n442 = local read "Report"() -> (w927:string)
                n443 = call "Reporting_datetime.vi"() -> ("String"=w925:string)  [unwired: 11 in]
                n444 = Concatenate Strings(w925, "\nSTATUS: ERROR TEST\n\n", w927) -> (w929:string)
                n445 = local write "Report"(w929) -> ()
              }
            }
            n446 = local read "Watchdog config"() -> (w920:T1)
            n447 = Merge Errors(w913, w911) -> (w912:errorcluster)
            n448 = call <vilib>:"Watchdog Configure.vi"("error in (no error)"=w911, "expiration actions"=w920, "timeout (1 sec)"=200.0) -> ("error out"=w921:errorcluster, "watchdogID"=w918:u64)  [unwired: 1 in, 2 out]
            n449 = flat-sequence {
              tunnel: [w939] -> w924
              tunnel: w921 -> [w934]
              tunnel: w912 -> [w952]
              tunnel: [w935] -> w922
              tunnel: w918 -> [w933]
              tunnel: [w932] -> w917
              tunnel: [w931] -> w916
              frame #0 {
                n450 = Get Date/Time In Seconds() -> (seconds since 1Jan1904=w946:timestamp)
                n451 = local read "Ultimo TEST"() -> (w947:timestamp)
                n452 = To Double Precision Float(number=w946) -> (double precision float=w948:dbl)
                n453 = Subtract(x=w948, y=3600.0) -> (x-y=w950:dbl)
                n454 = To Time Stamp(1:w950) -> (0:w951:timestamp)
                n455 = call <vilib>:"Watchdog Whack.vi"("error in (no error)"=w934, "reset watchdog after expire? (F)"=TRUE, "watchdogID in"=w933) -> ("error out"=w931:errorcluster, "watchdogID out"=w932:u64)  [unwired: 2 in, 1 out]
                n456 = In Range and Coerce(upper limit=w946, x=w947, lower limit=w951) -> (In Range?=w945:bool)  [unwired: 1 out]
                n457 = case shown="False" w945 {
                  tunnel: w952 -> [w962 w986]
                  tunnel: [w962 w986] -> w935
                  frame False {
                    n458 = local read "Timeout ruedas"() -> (w963:bool)
                    n459 = local read "Aviso no detección"() -> (w966:string)
                    n460 = local read "Aviso temperatura"() -> (w965:string)
                    n461 = case shown="True" w963 {
                      selector: w963 -> [_ w983]
                      tunnel: ["\r" w984] -> w961
                      frame False {
                      }
                      frame True {
                        w973 = "\n"
                        n462 = local read "Nº Ruedas 1"() -> (w980:i32)
                        n463 = local read "NºRuedas 2"() -> (w975:i32)
                        n464 = call "ErrorRuedas.vi"("Buffer Overflow"=w983) -> ("error out"=w985:errorcluster)
                        n465 = Number To Decimal String(number=w980) -> (decimal integer string=w978:string)  [unwired: 1 in]
                        n466 = Number To Decimal String(number=w975) -> (decimal integer string=w974:string)  [unwired: 1 in]
                        n467 = Concatenate Strings("Error Wheel sensors", "\n", "WS1 (wheels):", w978, w973, "WS2 (wheels):", w974, w973) -> (w976:string)
                        n468 = call "Error.vi"("Error con..."=w976, "error comunicacion 2"=w985) -> ("String"=w984:string)
                      }
                    }
                    n469 = local read "DC OK"() -> (w964:string)
                    n470 = call "Cabecera.vi"() -> ("String"=w971:string)
                    n471 = call "Adquisicion.vi"("Aviso no detección"=w966) -> ("String"=w970:string)
                    n472 = call "Temperatura.vi"("Aviso temperatura"=w965) -> ("String"=w969:string)
                    n473 = call "Fuente.vi"("DC OK"=w964) -> ("String"=w968:string)
                    n474 = call "FPGA.vi"("error out"=w962) -> ("String"=w967:string)
                    n475 = Get Date/Time In Seconds() -> (seconds since 1Jan1904=→"Ultimo TEST":timestamp)
                    n476 = Concatenate Strings(w971, w970, w969, w968, w967, w961) -> (w955:string)
                    n477 = local read "Report"() -> (w954:string)
                    n478 = Concatenate Strings(w955, w954) -> (w956:string)
                    n479 = local read "Max archivos"() -> (w957:u32)
                    n480 = local read "Path LOG"() -> (w960:path)
                    n481 = local read "LOG.txt"() -> (w958:path)
                    n482 = call "Saving_LOG.vi"("Path"=w958, "Report"=w956, "Report AURA"=w955, "Path Carpeta"=w960, "Nº Archivos Max"=w957) -> ("Report"=w959:string)  [unwired: 9 in, 1 out]
                    n483 = local write "Report"(w959) -> ()
                  }
                  frame True {
                  }
                }
                n484 = local read "Fallo fotocelula"() -> (w938:bool)
                n485 = local read "T fuera rango"() -> (w944:bool)
                n486 = Unbundle By Name(w935) -> ("status"=w936:bool)
                n487 = Compound Arithmetic op=OR(w936, w938) -> (w937:bool)
                n488 = local write "Reset del controlador"(w937) -> ()
                n489 = Select(t="UPS", s=w944, f="Espera") -> (s? t:f=w941:string)
                n490 = Select(t="Configuracion", s=w937, f=w941) -> (s? t:f=w939:string)
              }
            }
            n491 = call <vilib>:"Watchdog Clear.vi"("error in (no error)"=w916, "watchdogID in"=w917) -> ("error out"=w914:errorcluster)  [unwired: 5 in]
          }
          frame "Calibracion" {
            n492 = flat-sequence {
              tunnel: w1002 -> [w1787]
              tunnel: w1001 -> [w1786]
              tunnel: [w1787] -> w1000
              tunnel: [w1786] -> w999
              frame #0 {
                n493 = local read "Report"() -> (w1783:string)
                n494 = call "Reporting_datetime.vi"() -> ("String"=w1782:string)  [unwired: 11 in]
                n495 = Concatenate Strings(w1782, "\nSTATUS: CALIBRATION\n\n\n", w1783) -> (w1785:string)
                n496 = local write "Report"(w1785) -> ()
              }
            }
            n497 = for {
              N: 5 -> [_]
              shift-right: [w1041] -> w993
              shift-left: w1000 -> [w1043]
              shift-right: [w1040] -> w989
              shift-left: w999 -> [w1042]
              shift-right: [w1038] -> _
              shift-left: "Adquisicion" ("element") -> [w1039]
              shift-right: [w1037] -> _
              shift-left: _ -> [w1035]
              shift-right: [w1033] -> w988
              shift-left: "" -> [w1032]
              i -> [w1031]
              stop <- w1036 stop-if-true
              n498 = case shown="\"Acel_calib\"" w1039 {
                tunnel: w1043 -> [w1051 w1281 w1486 w1648 w1733]
                tunnel: w1042 -> [w1050 w1280 w1485 w1647 w1732]
                tunnel: [w1049 w1281 w1486 w1648 w1733] -> w1041
                tunnel: [w1048 w1280 w1485 w1647 w1732] -> w1040
                tunnel: ["Acel_calib" ("Concept") "Acel_frequency" ("Concept") "Acel_noise" ("Concept") "Acel_result" ("Concept") "Adquisicion" ("Concept")] -> w1038
                tunnel: [sgl[][] [] w1277 w1484 w1646 sgl[][] []] -> w1037
                tunnel: [TRUE w1276 w1483 w1643 FALSE] -> w1030
                tunnel: w1035 -> [_ _ w1474 w1649 w1743]
                tunnel: ["\n" w1274 w1481 w1639 w1731] -> w1034
                frame "Adquisicion", Default {
                  n499 = flat-sequence {
                    tunnel: w1050 -> [w1073]
                    tunnel: w1051 -> [w1074]
                    tunnel: [w1074] -> w1054
                    tunnel: [w1073] -> w1053
                    tunnel: [w1057] -> w1052
                    tunnel: w1054 -> [w1086]
                    tunnel: w1053 -> [w1085]
                    tunnel: w1052 -> [w1082]
                    tunnel: [w1084] -> w1049
                    tunnel: [w1083] -> w1048
                    frame #0 {
                      w1069 = "Calibration" ("element")
                      w1068 = "c"
                      n500 = Format Date/Time String(time format string (%c)="%Y-%m-%d-%H-%M-%S") -> (date/time string=w1060:string)  [unwired: 2 in]
                      n501 = for {
                        N: 1 -> [_]
                        shift-right: [w1075] -> w1055
                        shift-left: _ -> [w1076]
                        n502 = Add(x=w1076, y=0.001) -> (x+y=w1075:dbl)
                      }
                      n503 = Number To Fractional String(number=w1055) -> (F-format string=w1064:string)  [unwired: 3 out]
                      n504 = Search and Replace String(input string=w1064, search string="." ("replace string (\"\")")) -> (result string=w1062:string)  [unwired: 1 in, 8 out]
                      n505 = for {
                        N: 3 -> [_]
                        shift-right: [w1080] -> w1058
                        shift-left: w1062 -> [w1078]
                        n506 = Search and Replace String(input string=w1078, search string="0", offset=4 ("offset (0)")) -> (result string=w1080:string)  [unwired: 1 in, 7 out]
                      }
                      n507 = Concatenate Strings(w1058, "_" ("replace string (\"\")"), w1060) -> (w1057:string)
                      "date/time string 2" <- w1057
                      n508 = Build Array(w1068, w1069, w1057) -> (w1067:string[])
                      n509 = Build Array(w1068, w1069, w1057, "Calibration_LOG.txt" ("element")) -> (w1071:string[])
                      n510 = Array of Strings to Path(0:w1067) -> (2:w1066:path)  [unwired: 1 out]
                      "Folder" <- w1066
                      n511 = Array of Strings to Path(0:w1071) -> (2:→"calibration log":path)  [unwired: 1 out]
                      n512 = Create Folder(path (use dialog)=w1066) -> ()  [unwired: 2 in, 3 out]
                    }
                    frame #1 {
                      n513 = for {
                        N: 11 -> [_]
                        shift-right: [w1105] -> w1084
                        shift-left: w1086 -> [w1115]
                        shift-right: [w1108] -> w1083
                        shift-left: w1085 -> [w1114]
                        tunnel: w1082 -> [w1101]
                        i -> [w1111]
                        n514 = xnode "Invoke Method"("FPGA VI Reference In"=w1115, "error in"=w1114) -> ("FPGA VI Reference Out"=w1113:refnum<k20>, "error out"=w1112:errorcluster)  [unwired: 1 in]
                        n515 = Increment(x=w1111) -> (x+1=w1110:i32)
                        n516 = Number To Decimal String(number=w1110) -> (decimal integer string=w1109:string)  [unwired: 1 in]
                        n517 = flat-sequence {
                          tunnel: w1113 -> [w1126]
                          tunnel: w1112 -> [w1125]
                          tunnel: w1109 -> [w1124]
                          tunnel: [w1126] -> w1107
                          tunnel: [w1125] -> w1106
                          tunnel: [w1119] -> w1102
                          tunnel: w1101 -> [w1119]
                          tunnel: [w1118] -> w1088
                          tunnel: w1107 -> [w1134]
                          tunnel: w1106 -> [w1133]
                          tunnel: [w1134] -> w1104
                          tunnel: [w1133] -> w1103
                          tunnel: w1102 -> [w1131]
                          tunnel: [w1131] -> w1100
                          tunnel: [w1130] -> w1089
                          tunnel: w1088 -> [w1130]
                          tunnel: w1104 -> [w1174]
                          tunnel: w1103 -> [w1173]
                          tunnel: w1100 -> [w1152]
                          tunnel: [w1172] -> w1099
                          tunnel: [w1171] -> w1098
                          tunnel: [w1145] -> w1097
                          tunnel: [w1144] -> w1096
                          tunnel: [w1143] -> w1095
                          tunnel: [w1142] -> w1094
                          tunnel: w1089 -> [w1135]
                          tunnel: w1099 -> [w1201]
                          tunnel: w1098 -> [w1202]
                          tunnel: w1097 -> [w1198]
                          tunnel: w1096 -> [w1197]
                          tunnel: w1095 -> [w1196]
                          tunnel: w1094 -> [w1195]
                          tunnel: [w1200] -> w1093
                          tunnel: [w1192] -> w1092
                          tunnel: [w1189] -> w1091
                          tunnel: [w1188] -> w1090
                          tunnel: [w1267] -> w1108
                          tunnel: [w1268] -> w1105
                          tunnel: w1093 -> [w1270]
                          tunnel: w1092 -> [w1269]
                          tunnel: w1091 -> [w1265]
                          tunnel: w1090 -> [w1264]
                          frame #0 {
                            w1116 = dbl[] [] ("mean")
                            n518 = local read "Report"() -> (w1121:string)
                            n519 = local write "mean"(w1116) -> ()
                            n520 = local write "median"(w1116) -> ()
                            n521 = local write "max"(w1116) -> ()
                            n522 = local write "min"(w1116) -> ()
                            n523 = local write "Value to compare"(w1116) -> ()
                            n524 = Concatenate Strings("\nAcquiring file: ", w1124, "/11\n" ("string"), w1121) -> (w1120:string)
                            n525 = for {
                              N: 1 -> [_]
                              shift-right: [w1127] -> w1118
                              shift-left: _ -> [w1128]
                              n526 = Add(x=w1128, y=0.001) -> (x+y=w1127:dbl)
                            }
                            n527 = local write "Report"(w1120) -> ()
                          }
                          frame #1 {
                            n528 = Wait (ms)(milliseconds to wait=u32 1000) -> ()  [unwired: 1 out]
                          }
                          frame #2 {
                            n529 = local read "Frecuencia de muestreo y módulo CRIO"() -> (w1170:T2)
                            n530 = local read "Frecuencia de muestreo (Hz)"() -> (w1168:dbl)
                            n531 = Number To Fractional String(number=w1135) -> (F-format string=w1149:string)  [unwired: 3 out]
                            n532 = local read "Escaneos de la FIFO por canal"() -> (w1167:u32)
                            n533 = xnode "Read/Write Control"("FPGA VI Reference In"=w1174, "error in"=w1173, "Fotocélula"=TRUE ("Adquirir")) -> ("FPGA VI Reference Out"=w1178:refnum<k20>, "error out"=w1177:errorcluster)
                            n534 = local read "Nº de acelerómetros"() -> (w1165:i32)
                            n535 = local read "Count(mSec)"() -> (w1169:u32)
                            n536 = local read "Nº inductivos"() -> (w1166:i32)
                            n537 = Search and Replace String(input string=w1149, search string="." ("replace string (\"\")")) -> (result string=w1147:string)  [unwired: 1 in, 8 out]
                            n538 = for {
                              N: 3 -> [_]
                              shift-right: [w1186] -> w1150
                              shift-left: w1147 -> [w1184]
                              n539 = Search and Replace String(input string=w1184, search string="0", offset=4 ("offset (0)")) -> (result string=w1186:string)  [unwired: 1 in, 7 out]
                            }
                            n540 = xnode "Read/Write Control"("FPGA VI Reference In"=w1178, "error in"=w1177, "Data Rate"=w1170, "Digital?"=TRUE, "Count(mSec)"=w1169) -> ("FPGA VI Reference Out"=w1180:refnum<k20>, "error out"=w1179:errorcluster)
                            n541 = Format Date/Time String(time format string (%c)="%Y-%m-%d-%H-%M-%S") -> (date/time string=w1151:string)  [unwired: 2 in]
                            n542 = Add(x=w1166, y=w1165) -> (x+y=w1164:i32)
                            n543 = call "DMACalc.vi"("Number of Channels"=w1164, "Number of Samples"=w1167, "Rate (Hz)"=w1168) -> ("Block Size"=w1144:u32, "Time to Acquire Block (ms)"=w1145:i32, "Host Buffer Size"=w1163:u32)  [unwired: 6 in]
                            n544 = xnode "Invoke Method"("FPGA VI Reference In"=w1180, "error in"=w1179, "Requested Depth"=w1163) -> ("FPGA VI Reference Out"=w1182:refnum<k20>, "error out"=w1181:errorcluster)  [unwired: 1 out]
                            n545 = Concatenate Strings(w1150, "_" ("replace string (\"\")"), w1151, ".bin" ("string")) -> (w1158:string)
                            n546 = Build Array("c", "Calibration" ("element"), w1152, w1158) -> (w1157:string[])
                            n547 = xnode "Invoke Method"("FPGA VI Reference In"=w1182, "error in"=w1181) -> ("FPGA VI Reference Out"=w1172:refnum<k20>, "error out"=w1171:errorcluster)
                            n548 = local read "Report"() -> (w1137:string)
                            n549 = Array of Strings to Path(0:w1157) -> (2:w1138:path)  [unwired: 1 out]
                            n550 = Path To String(path=w1138) -> (string=w1141:string)
                            n551 = Get Date/Time In Seconds() -> (seconds since 1Jan1904=→"Inicio pasada 2":timestamp)
                            n552 = Concatenate Strings("\nFile created: ", w1141, "\n", w1137) -> (w1136:string)
                            n553 = Open/Create/Replace File(file path (use dialog)=w1138, operation (0:open)=T4."replace or create", access (0:read/write)=enum16{"read/write", "read-only", "write-only"}."read/write", disable buffering (F)=TRUE) -> (refnum out=w1143:refnum<file>, error out=w1142:errorcluster)  [unwired: 1 in, 2 out]
                            n554 = local write "Report"(w1136) -> ()
                          }
                          frame #3 {
                            n555 = while "Data Acquisition" {
                              tunnel: w1201 -> [w1227]
                              shift-right: [w1234] -> _
                              shift-left: u32 0 ("t") -> [w1230]
                              tunnel: w1198 -> [w1235]
                              tunnel: w1197 -> [w1233]
                              shift-right: [w1236] -> w1192
                              shift-left: w1202 -> [w1226]
                              tunnel: [w1231] -> w1200
                              tunnel: w1196 -> [w1216]
                              tunnel: [w1217] -> w1189
                              shift-right: [w1215] -> w1188
                              shift-left: w1195 -> [w1224]
                              stop <- w1232 stop-if-true
                              # "Detector de presencia"
                              # "Mide el tiempo de paso del tren y con ello se puede calcular\nla velocidad la unidad"
                              n556 = xnode "Invoke Method"("FPGA VI Reference In"=w1227, "error in"=w1226, "Number of Elements"=w1230, "Timeout (ms)"=0) -> ("FPGA VI Reference Out"=w1214:refnum<k20>, "error out"=w1213:errorcluster, "Data"=w1225:fxp<+/-,24,4>[], "Elements Remaining"=w1228:u32)
                              n557 = case "Data Ready" shown="Default" w1230 {
                                tunnel: w1235 -> [w1241 _]
                                tunnel: [w1240 u32 0 ("t")] -> w1234
                                tunnel: w1233 -> [w1242 _]
                                tunnel: w1228 -> [w1239 _]
                                tunnel: w1225 -> [_ w1252]
                                tunnel: w1224 -> [w1238 w1254]
                                tunnel: [w1238 w1253] -> w1215
                                tunnel: w1216 -> [w1237 w1251]
                                tunnel: [w1237 w1250] -> w1217
                                frame 0 {
                                n558 = Greater Or Equal?(x=w1239, y=w1242) -> (x >= y?=w1243:bool)
                                n559 = case shown="False" w1243 {
                                tunnel: [u32 0 ("Block Size") w1247] -> w1240
                                tunnel: [w1246 0 ("t")] -> w1244
                                tunnel: w1241 -> [w1246 _]
                                tunnel: w1242 -> [_ w1247]
                                frame False {
                                }
                                frame True {
                                }
                                }
                                n560 = call "WaitMinTimeBetweenCall.vi"("Minimum ms between calls"=w1244) -> ()  [unwired: 2 in]
                                }
                                frame Default {
                                n561 = To Single Precision Float(number=w1252) -> (single precision float=w1249:sgl[])
                                n562 = Write to Binary File(file (use dialog)=w1251, data=w1249, error in=w1254, 5:FALSE ("prepend array or string size? (T)"), 9:T5."little-endian" ("byte order (0:big-endian, network order)")) -> (refnum out=w1250:refnum<file>, error out=w1253:errorcluster)  [unwired: 2 out]
                                }
                              }
                              n563 = local read "Inicio pasada 2"() -> (w1205:timestamp)
                              n564 = Get Date/Time In Seconds() -> (seconds since 1Jan1904=w1206:timestamp)
                              n565 = xnode ("CheckLate")("FPGA VI Reference In"=w1214, "error in"=w1213) -> ("FPGA VI Reference Out"=w1208:refnum<k20>, "error out"=w1222:errorcluster, "Buffer Underflow"=w1203:bool, "Buffer Overflow"=w1204:bool)
                              n566 = To Double Precision Float(number=w1206) -> (double precision float=w1211:dbl)
                              n567 = To Double Precision Float(number=w1205) -> (double precision float=w1212:dbl)
                              n568 = Subtract(x=w1211, y=w1212) -> (x-y=w1219:dbl)
                              "Acquiring time" <- w1219
                              n569 = local write "Buffer Overflow"(w1204) -> ()
                              n570 = local write "Buffer Underflow"(w1203) -> ()
                              n571 = Greater?(x=w1219, y=1.0 ("Tiempo de adquisición")) -> (0:w1210:bool)
                              n572 = call "ErrorOverFlow.vi"("Buffer Overflow"=w1204) -> ("error out"=w1220:errorcluster)
                              n573 = call "ErrorUnderFlow.vi"("Buffer Overflow"=w1203) -> ("error out"=w1221:errorcluster)
                              n574 = Merge Errors(w1222, w1221, w1220) -> (w1209:errorcluster)
                              n575 = Unbundle By Name(w1215) -> ("status"=w1218:bool)
                              n576 = Unbundle By Name(w1209) -> ("status"=w1223:bool)
                              n577 = Compound Arithmetic op=OR(w1223, w1210, w1218) -> (w1232:bool)
                              n578 = case "Flush" shown="True" w1232 {
                                tunnel: w1208 -> [w1258 w1263]
                                tunnel: w1209 -> [w1259 w1262]
                                tunnel: [w1259 w1261] -> w1236
                                tunnel: [w1258 w1260] -> w1231
                                frame False {
                                }
                                frame True {
                                n579 = xnode "Invoke Method"("FPGA VI Reference In"=w1263, "error in"=w1262) -> ("FPGA VI Reference Out"=w1260:refnum<k20>, "error out"=w1261:errorcluster)
                                }
                              }
                            }
                            n580 = call "Reporting_error.vi"("error out 2"=w1192, "Concept"="FPGA ") -> ("Reporting"=w1194:string)  [unwired: 1 in]
                            n581 = local read "Report"() -> (w1191:string)
                            n582 = Concatenate Strings(w1194, w1191) -> (w1193:string)
                            n583 = local write "Report"(w1193) -> ()
                          }
                          frame #4 {
                            n584 = xnode "Read/Write Control"("FPGA VI Reference In"=w1270, "error in"=w1269, "Stop"=TRUE) -> ("FPGA VI Reference Out"=w1271:refnum<k20>, "error out"=w1272:errorcluster)
                            n585 = Close File(refnum=w1265, error in=w1264) -> ()  [unwired: 2 out]
                            n586 = xnode "Invoke Method"("FPGA VI Reference In"=w1271, "error in"=w1272) -> ("FPGA VI Reference Out"=w1268:refnum<k20>, "error out"=w1267:errorcluster)
                          }
                        }
                      }
                    }
                  }
                }
                frame "Acel_calib" {
                  n587 = local read "Folder"() -> (w1283:path)
                  n588 = local read "Frecuencia de muestreo (Hz)"() -> (w1289:dbl)
                  n589 = local read "Nº de acelerómetros"() -> (w1284:i32)
                  n590 = local read "Nº inductivos"() -> (w1285:i32)
                  n591 = local read "Pattern frequency (Hz)"() -> (w1290:dbl)
                  n592 = call <vilib>:"Recursive File List.vi"("Folder Path"=w1283) -> ("All Files in Dir"=w1288:path[])  [unwired: 6 in, 4 out]
                  n593 = Array Size(array=w1288) -> (size(s)=→"Nº meas":i32)
                  n594 = Add(x=w1285, y=w1284) -> (x+y=w1287:i32)
                  n595 = flat-sequence {
                    tunnel: w1288 -> [w1300]
                    tunnel: [w1300] -> w1296
                    tunnel: [w1299] -> w1295
                    tunnel: w1287 -> [w1299]
                    tunnel: [w1298] -> w1294
                    tunnel: w1289 -> [w1298]
                    tunnel: [w1297] -> w1293
                    tunnel: w1290 -> [w1297]
                    tunnel: [w1307] -> w1292
                    tunnel: [w1306] -> w1291
                    tunnel: w1296 -> [w1308]
                    tunnel: w1295 -> [w1305]
                    tunnel: w1294 -> [w1304]
                    tunnel: w1293 -> [w1303]
                    tunnel: [w1302] -> w1273
                    tunnel: w1292 -> [w1420]
                    tunnel: w1291 -> [w1409]
                    tunnel: [w1401] -> w1277
                    tunnel: [TRUE] -> w1276
                    tunnel: [w1435] -> w1274
                    tunnel: [w1410] -> w1275
                    tunnel: w1273 -> [w1405]
                    frame #0 {
                      "Valid\nindex" <- i32[] []
                    }
                    frame #1 {
                      n596 = for {
                        tunnel: w1308 -> [w1330] mode=indexing
                        tunnel: [w1320] -> w1307 mode=indexing
                        tunnel: [w1310] -> w1306 mode=indexing
                        tunnel: w1305 -> [w1318]
                        tunnel: w1304 -> [w1317]
                        tunnel: w1303 -> [w1316]
                        tunnel: [w1309] -> w1302 mode=indexing
                        n597 = Read from Binary File(5:sgl 1.25, 9:T5."little-endian" ("byte order (0:big-endian, network order)"), 10:-1 ("count (1)"), 11:w1330) -> (2:w1331:sgl[])  [unwired: 1 in, 4 out]
                        n598 = case shown="10" w1318 {
                          tunnel: [w1348 w1361 w1371] -> w1310
                          tunnel: w1331 -> [w1349 w1359 w1372]
                          frame 9, Default {
                            n599 = Decimate 1D Array(w1349) -> (w1350:sgl[], w1358:sgl[], w1357:sgl[], w1353:sgl[], w1352:sgl[], w1354:sgl[], w1355:sgl[], w1356:sgl[], w1351:sgl[])
                            n600 = Build Array(w1350, w1358, w1357, w1353, w1352, w1354, w1355, w1356, w1351) -> (w1348:sgl[][])
                          }
                          frame 10 {
                            n601 = Decimate 1D Array(w1359) -> (w1360:sgl[], w1370:sgl[], w1369:sgl[], w1365:sgl[], w1364:sgl[], w1366:sgl[], w1367:sgl[], w1368:sgl[], w1363:sgl[], w1362:sgl[])
                            n602 = Build Array(w1360, w1370, w1369, w1365, w1364, w1366, w1367, w1368, w1363, w1362) -> (w1361:sgl[][])
                          }
                          frame 5 {
                            n603 = Decimate 1D Array(w1372) -> (w1373:sgl[], w1377:sgl[], w1376:sgl[], w1375:sgl[], w1374:sgl[])
                            n604 = Build Array(w1373, w1377, w1376, w1375, w1374) -> (w1371:sgl[][])
                          }
                        }
                        n605 = for {
                          tunnel: w1310 -> [w1380] mode=indexing
                          tunnel: [w1383] -> w1327 mode=indexing
                          tunnel: w1317 -> [w1382]
                          tunnel: w1316 -> [w1381]
                          n606 = call-poly <vilib>:"Basic Averaged DC-RMS.vi"("signal in"=w1380) -> ("DC value"=w1393:dbl)  [unwired: 7 in, 3 out]
                          n607 = Array Size(array=w1380) -> (size(s)=→"size(s) 3":i32)
                          n608 = Subtract(x=w1380, y=w1393) -> (x-y=w1389:dbl[])
                          n609 = Divide(x=w1382, y=w1381) -> (x/y=w1390:dbl)
                          n610 = Array Size(array=w1389) -> (size(s)=w1391:i32)
                          n611 = Subtract(x=w1391, y=w1390) -> (x-y=w1392:dbl)
                          n612 = for {
                            N: w1392 -> [_]
                            tunnel: w1390 -> [w1395]
                            tunnel: [w1398] -> w1378 mode=indexing
                            tunnel: w1389 -> [w1397]
                            i -> [w1396]
                            n613 = Array Subset(array=w1397, index=w1396, length=w1395) -> (w1394:dbl[])
                            n614 = call-poly <vilib>:"RMS.vi"("X"=w1394) -> ("rms value"=w1398:dbl)  [unwired: 1 out]
                          }
                          n615 = Greater?(x=w1378, y=0.004 ("threshold y")) -> (0:w1387:bool[])
                          n616 = Search 1D Array(1D array=w1387, element=TRUE) -> (index of element=w1385:i32)  [unwired: 1 in]
                          n617 = Not Equal?(x=w1385, y=-1) -> (x != y?=w1383:bool)
                        }
                        n618 = Array Size(array=w1310) -> (size(s)=→"size(s)":i32[])
                        n619 = while {
                          tunnel: w1327 -> [w1347]
                          shift-right: [w1339] -> _
                          shift-left: 0 ("index of element") -> [w1344]
                          shift-right: [w1340] -> w1319
                          shift-left: 0 ("index of element") -> [w1341]
                          tunnel: [w1338] -> w1315 mode=indexing
                          i -> [w1342]
                          stop <- w1345 stop-if-true
                          n620 = Add(x=w1341, y=w1342) -> (x+y=w1340:i32)
                          n621 = Search 1D Array(1D array=w1347, element=TRUE, start index (0)=w1344) -> (index of element=w1338:i32)
                          n622 = Equal?(x=w1338, y=-1) -> (x = y?=w1345:bool)
                          n623 = Increment(x=w1338) -> (x+1=w1339:i32)
                        }
                        n624 = Delete From Array(array=w1315, length=1) -> (array with subset deleted=w1314:i32[])  [unwired: 1 in, 1 out]
                        n625 = Array Size(array=w1314) -> (size(s)=w1323:i32)
                        n626 = Equal?(x=w1319, y=1) -> (x = y?=w1322:bool)
                        n627 = Equal?(x=w1323, y=1) -> (x = y?=w1321:bool)
                        n628 = And(x=w1321, y=w1322) -> (x .and. y?=w1320:bool)
                        n629 = case shown="True" w1320 {
                          tunnel: w1314 -> [_ w1337]
                          frame False {
                          }
                          frame True {
                            n630 = local read "Valid\nindex"() -> (w1335:i32[])
                            n631 = Insert Into Array(array=w1335, new element=w1337) -> (w1336:i32[])  [unwired: 1 in]
                            n632 = local write "Valid\nindex"(w1336) -> ()
                          }
                        }
                        n633 = Array Size(array=w1310) -> (size(s)=w1312:i32[])
                        n634 = Index Array(array=w1312, index=1) -> (element=w1309:i32)
                      }
                    }
                    frame #2 {
                      w1419 = 0 ("index of element")
                      (unwired) 0 ("index of element")
                      n635 = local read "Valid\nindex"() -> (w1425:i32[])
                      n636 = Array Max & Min(array=w1405) -> (min value=w1402:i32)  [unwired: 3 out]
                      n637 = Sort 1D Array(array=w1425) -> (sorted array=w1421:i32[])
                      "sorted array" <- w1421
                      n638 = Decrement(x="Accelerometer") -> (x-1=w1400:i32)
                      n639 = for {
                        tunnel: w1421 -> [w1456] mode=indexing
                        shift-right: [w1456] -> _
                        shift-left: -1 ("y") -> [w1457]
                        tunnel: [w1456] -> w1430 mode=indexing if=w1455
                        shift-right: [w1452] -> _
                        shift-left: 0 ("y") -> [w1453]
                        tunnel: [w1452] -> w1428 mode=indexing
                        n640 = Not Equal?(x=w1456, y=w1457) -> (x != y?=w1455:bool)
                        n641 = Increment(x=w1453) -> (x+1=w1454:i32)
                        n642 = Select(t=1 ("y"), s=w1455, f=w1454) -> (s? t:f=w1452:i32)
                      }
                      "Array" <- w1430
                      "Array 3" <- w1428
                      n643 = Delete From Array(array=w1409, index (dim 1)=w1400) -> (deleted portion=w1403:sgl[][])  [unwired: 3 in, 1 out]
                      n644 = for {
                        tunnel: w1420 -> [w1462] mode=indexing
                        shift-right: [w1461] -> _
                        shift-left: w1409 -> [w1463]
                        shift-right: [w1458] -> _
                        shift-left: 0 ("index of element") -> [w1459]
                        i -> [w1460]
                        n645 = case shown="False" w1462 {
                          tunnel: w1463 -> [w1469 w1471]
                          tunnel: [w1468 w1471] -> w1461
                          tunnel: w1460 -> [w1467 _]
                          tunnel: w1459 -> [w1464 w1470]
                          tunnel: [w1465 w1470] -> w1458
                          frame False {
                            n646 = Subtract(x=w1467, y=w1464) -> (x-y=w1466:i32)
                            n647 = Delete From Array(array=w1469, index (dim 0)=w1466) -> (array with subset deleted=w1468:sgl[][][])  [unwired: 3 in, 1 out]
                            n648 = Increment(x=w1464) -> (x+1=w1465:i32)
                          }
                          frame True {
                          }
                        }
                      }
                      n649 = Array Subset(array=w1403, index (col)=0 ("index"), length (col)=w1402) -> (w1401:sgl[][])  [unwired: 2 in]
                      n650 = Array Max & Min(array=w1428) -> (max value=→"max value":i32, max index (indices)=w1426:i32)  [unwired: 2 out]
                      "max index(es)" <- w1426
                      n651 = Index Array(array=w1421, index=w1426) -> (element=w1410:i32)
                      "element" <- w1410
                      n652 = local read "Frecuencia de muestreo (Hz)"() -> (w1408:dbl)
                      n653 = Equal?(x=w1425, y=w1410) -> (x = y?=w1423:bool[])
                      n654 = Boolean To (0,1)(Boolean=w1423) -> (0, 1=w1422:i16[])
                      n655 = Add Array Elements(numeric array=w1422) -> (sum=w1414:i16)
                      n656 = Equal?(x=w1410, y=w1419) -> (x = y?=w1417:bool)
                      n657 = Equal?(x=w1419, y=w1414) -> (x = y?=w1416:bool)
                      n658 = Increment(x=w1410) -> (x+1=w1424:i32)
                      n659 = local read "Nº meas"() -> (w1436:i32)
                      n660 = Not And(1:w1416, 2:w1417) -> (0:w1415:bool)
                      n661 = for {
                        tunnel: w1401 -> [w1450] mode=indexing
                        tunnel: w1408 -> [w1448]
                        tunnel: [w1447] -> w1407 mode=indexing
                        n662 = Reciprocal(x=w1448) -> (1/x=w1449:dbl)
                        n663 = Bundle By Name("Y"=w1450, "dt"=w1449) -> (w1447:waveform(sgl))  [unwired: 1 in]
                      }
                      n664 = Number To Decimal String(number=w1424) -> (decimal integer string=w1412:string)  [unwired: 1 in]
                      n665 = Select(t=w1412, s=w1415, f=" NONE ") -> (s? t:f=w1413:string)
                      n666 = Number To Decimal String(number=w1414) -> (decimal integer string=w1442:string)  [unwired: 1 in]
                      n667 = Number To Decimal String(number=w1436) -> (decimal integer string=w1440:string)  [unwired: 1 in]
                      n668 = Divide(x=w1414, y=w1436) -> (x/y=w1438:dbl)
                      n669 = for {
                        tunnel: w1407 -> [w1446] mode=indexing
                        tunnel: [w1443] -> w1406 mode=concatenating
                        n670 = call "Convert to Dynamic Data"("Waveform"=w1446) -> ("Dynamic Data Type"=w1445:dynamicdata)  [unwired: 3 in]
                        n671 = call "Tone Measurements"("Signals"=w1445) -> ("Frequency"=w1444:dynamicdata)  [unwired: 9 in, 1 out]
                        n672 = call "Convert from Dynamic Data"("Dynamic Data Type"=w1444) -> ("Array"=w1443:dbl[])  [unwired: 3 in]
                      }
                      "Frequency" <- w1406
                      n673 = Greater?(x=w1438, y=0.6) -> ()  [unwired: 1 out]
                      n674 = Concatenate Strings("\nACCELEROMETER DETECTOR:\n\nAccelerometer detected: ", w1413, " \nAccelerometer detected in  ", w1442, " of ", w1440, " measurements\n------------------------------------------------------------------------------------------------------------------------------------------------") -> (w1435:string)
                    }
                  }
                  n675 = local read "Report"() -> (w1278:string)
                  n676 = Concatenate Strings(w1274, w1278) -> (w1279:string)
                  n677 = local write "Report"(w1279) -> ()
                  "Accel.detected" <- w1275
                }
                frame "Acel_frequency" {
                  n678 = local read "Low cutoff freq"() -> (w1476:dbl)
                  n679 = local read "Frequency"() -> (w1477:dbl[])
                  n680 = local read "Frecuencia de muestreo (Hz)"() -> (w1479:dbl)
                  n681 = for {
                    tunnel: w1474 -> [w1510] mode=indexing
                    tunnel: w1479 -> [w1508]
                    tunnel: [w1507] -> w1478 mode=indexing
                    n682 = Reciprocal(x=w1508) -> (1/x=w1509:dbl)
                    n683 = Bundle By Name("Y"=w1510, "dt"=w1509) -> (w1507:waveform(sgl))  [unwired: 1 in]
                  }
                  "Waveform Graph" <- w1478
                  n684 = local read "Pattern frequency (Hz)"() -> (w1480:dbl)
                  n685 = Less?(x=w1477, y=w1476) -> (x < y?=w1472:bool[])
                  n686 = for {
                    tunnel: w1472 -> [w1497] mode=indexing
                    shift-right: [w1496] -> w1473
                    shift-left: w1474 -> [w1498]
                    shift-right: [w1493] -> _
                    shift-left: 0 ("index of element") -> [w1494]
                    i -> [w1495]
                    n687 = case shown="False" w1497 {
                      tunnel: w1498 -> [w1504 w1506]
                      tunnel: [w1503 w1506] -> w1496
                      tunnel: w1495 -> [w1502 _]
                      tunnel: w1494 -> [w1499 w1505]
                      tunnel: [w1500 w1505] -> w1493
                      frame False {
                        n688 = Subtract(x=w1502, y=w1499) -> (x-y=w1501:i32)
                        n689 = Delete From Array(array=w1504, index (row)=w1501) -> (array with subset deleted=w1503:sgl[][])  [unwired: 2 in, 1 out]
                        n690 = Increment(x=w1499) -> (x+1=w1500:i32)
                      }
                      frame True {
                      }
                    }
                  }
                  n691 = flat-sequence {
                    tunnel: w1473 -> [w1517]
                    tunnel: w1479 -> [w1514]
                    tunnel: w1480 -> [w1511]
                    tunnel: [w1519] -> w1492
                    tunnel: [w1513] -> w1491
                    tunnel: [w1512] -> w1490
                    tunnel: [w1511] -> w1489
                    tunnel: w1492 -> [w1596]
                    tunnel: w1491 -> [w1578]
                    tunnel: w1490 -> [w1595]
                    tunnel: w1489 -> [w1594]
                    tunnel: [w1596] -> w1484
                    tunnel: [w1580] -> w1481
                    tunnel: [w1579] -> w1483
                    tunnel: [w1578] -> _
                    frame #0 {
                      n692 = for {
                        tunnel: w1517 -> [w1569] mode=indexing
                        tunnel: w1514 -> [w1568]
                        tunnel: w1511 -> [w1564]
                        tunnel: [w1545] -> w1513 mode=indexing
                        tunnel: [w1539] -> w1512 mode=indexing
                        n693 = Reciprocal(x=w1568) -> (1/x=w1570:dbl)
                        n694 = Bundle By Name("Y"=w1569, "dt"=w1570) -> (w1567:waveform(sgl))  [unwired: 1 in]
                        n695 = call-poly <vilib>:"FFT Spectrum (Mag-Phase).vi"("time signal"=w1567) -> ("magnitude"=w1566:cluster{"f0":dbl, "df":dbl, "magnitude":dbl[]})  [unwired: 6 in, 4 out]
                        n696 = Unbundle By Name(w1566) -> ("magnitude"=w1558:dbl[], "df"=w1540:dbl)
                        n697 = Multiply(x=1.03, y=w1564) -> (x*y=w1561:dbl)
                        n698 = Multiply(x=w1564, y=0.97 ("x")) -> (x*y=w1562:dbl)
                        n699 = Divide(x=w1562, y=w1540) -> (x/y=w1559:dbl)
                        n700 = Divide(x=w1561, y=w1540) -> (x/y=w1556:dbl)
                        n701 = Array Max & Min(array=w1558) -> (max value=w1551:dbl, max index (indices)=w1541:i32)  [unwired: 2 out]
                        n702 = Array Size(array=w1558) -> (size(s)=w1557:i32)
                        n703 = Multiply(x=w1541, y=w1540) -> (x*y=w1539:dbl)
                        n704 = Subtract(x=w1557, y=w1556) -> (x-y=w1555:dbl)
                        n705 = In Range and Coerce(upper limit=w1561, x=w1539, lower limit=w1562) -> (In Range?=w1544:bool)  [unwired: 1 out]
                        n706 = Array Subset(array=w1558, index=w1556, length=w1555) -> (w1554:dbl[])
                        n707 = Array Subset(array=w1558, index=0, length=w1559) -> (w1553:dbl[])
                        n708 = Array Max & Min(array=w1554) -> (max value=w1552:dbl)  [unwired: 3 out]
                        n709 = Array Max & Min(array=w1553) -> (max value=w1550:dbl)  [unwired: 3 out]
                        n710 = Divide(x=w1551, y=w1550) -> (x/y=w1548:dbl)
                        n711 = Divide(x=w1551, y=w1552) -> (x/y=w1549:dbl)
                        n712 = Greater?(x=w1549, y=3.0) -> (0:w1543:bool)
                        n713 = Greater?(x=w1548, y=3.0) -> (0:w1542:bool)
                        n714 = Compound Arithmetic op=AND(w1544, w1543, w1542) -> (w1545:bool)
                      }
                      n715 = for {
                        shift-right: [w1526] -> w1519
                        shift-left: w1517 -> [w1527]
                        tunnel: w1513 -> [w1525] mode=indexing
                        shift-right: [w1522] -> _
                        shift-left: 0 ("index of element") -> [w1523]
                        shift-right: [w1520] -> w1516
                        shift-left: w1512 -> [w1521]
                        i -> [w1524]
                        n716 = case shown="True" w1525 {
                          tunnel: w1527 -> [w1535 w1538]
                          tunnel: [w1534 w1538] -> w1526
                          tunnel: w1524 -> [w1533 _]
                          tunnel: w1523 -> [w1532 w1537]
                          tunnel: [w1531 w1537] -> w1522
                          tunnel: w1521 -> [w1530 w1536]
                          tunnel: [w1528 w1536] -> w1520
                          frame False {
                            n717 = Subtract(x=w1533, y=w1532) -> (x-y=w1529:i32)
                            n718 = Delete From Array(array=w1535, index (row)=w1529) -> (array with subset deleted=w1534:sgl[][])  [unwired: 2 in, 1 out]
                            n719 = Increment(x=w1532) -> (x+1=w1531:i32)
                            n720 = Delete From Array(array=w1530, index=w1529) -> (array with subset deleted=w1528:dbl[])  [unwired: 1 in, 1 out]
                          }
                          frame True {
                          }
                        }
                      }
                      n721 = call <vilib>:"Std Deviation and Variance.vi"("X"=w1516) -> ("mean"=→"Mean\nfrequency":dbl)  [unwired: 1 in, 2 out]
                    }
                    frame #1 {
                      w1575 = "\r"
                      n722 = for {
                        tunnel: w1578 -> [w1604] mode=indexing
                        tunnel: w1595 -> [w1623] mode=indexing
                        tunnel: w1594 -> [w1622]
                        tunnel: [w1605] -> w1592 mode=indexing
                        shift-right: [w1599] -> w1590
                        shift-left: 0 -> [w1600]
                        i -> [w1625]
                        n723 = Increment(x=w1625) -> (x+1=w1624:i32)
                        n724 = Select(t=1, s=w1604, f=0) -> (s? t:f=w1601:i32)
                        n725 = Divide(x=w1623, y=w1622) -> (x/y=w1620:dbl)
                        n726 = Select(t="TRUE", s=w1604, f="FALSE") -> (s? t:f=w1614:string)
                        n727 = Number To Decimal String(number=w1624) -> (decimal integer string=w1617:string)  [unwired: 1 in]
                        n728 = Number To Fractional String(number=w1623, precision (6)=i16 2) -> (F-format string=w1611:string)  [unwired: 2 in]
                        n729 = Add(x=w1601, y=w1600) -> (x+y=w1599:i32)
                        n730 = Greater Than 0?(x=w1620) -> (x > 0?=w1621:bool)
                        n731 = case shown="True" w1621 {
                          tunnel: w1620 -> [w1633 w1635]
                          tunnel: [w1629 w1637] -> w1619
                          tunnel: ["-" " "] -> w1609
                          frame False {
                            n732 = Subtract(x=1.0, y=w1633) -> (x-y=w1631:dbl)
                            n733 = Multiply(x=100.0, y=w1631) -> (x*y=w1629:dbl)
                          }
                          frame True {
                            n734 = Decrement(x=w1635) -> (x-1=w1636:dbl)
                            n735 = Multiply(x=100.0, y=w1636) -> (x*y=w1637:dbl)
                          }
                        }
                        n736 = Number To Fractional String(number=w1619, precision (6)=i16 2) -> (F-format string=w1608:string)  [unwired: 2 in]
                        n737 = Concatenate Strings("\n\nMeasurement: ", w1617, "\r", "Frequency valid: ", w1614, "\r", "Frequency: ", w1611, ", ", w1609, w1608, " % of error in frequency", "\r") -> (w1605:string)
                      }
                      n738 = Array Size(array=w1578) -> (size(s)=w1589:i32)
                      n739 = Number To Decimal String(number=w1589) -> (decimal integer string=w1584:string)  [unwired: 1 in]
                      n740 = Number To Decimal String(number=w1590) -> (decimal integer string=w1576:string)  [unwired: 1 in]
                      n741 = Divide(x=w1590, y=w1589) -> (x/y=w1573:dbl)
                      n742 = Greater?(x=w1573, y=0.8) -> (0:w1579:bool)
                      n743 = Multiply(x=100.0, y=w1573) -> (x*y=w1572:dbl)
                      n744 = Number To Fractional String(number=w1572, precision (6)=i16 2) -> (F-format string=w1583:string)  [unwired: 2 in]
                      n745 = Select(t="OK\n------------------------------------------------------------------------", s=w1579, f="FAIL (REPEAT ACEL CALIBRATION)\n------------------------------------------------------------------------") -> (s? t:f=w1581:string)
                      n746 = Concatenate Strings("FREQUENCY TEST:\n \n- MEASUREMENT OK IF +/- 5% FREQ PATTERN\n\n- FREQUENCY ANALYSYS MORE THAN 80% OF THE MEASUREMENTS INSIDE OF THE RANGE\n", w1592, w1575, w1575, w1576, " measurements OK of ", w1584, " , ", w1583, " %\n\nFREQUENCY ANALYSIS: ", w1581) -> (w1580:string)
                    }
                  }
                  n747 = local read "Report"() -> (w1488:string)
                  n748 = Concatenate Strings(w1481, w1488) -> (w1487:string)
                  n749 = local write "Report"(w1487) -> ()
                }
                frame "Acel_noise" {
                  n750 = local read "Frecuencia de muestreo (Hz)"() -> (w1642:dbl)
                  n751 = local read "Pattern frequency (Hz)"() -> (w1641:dbl)
                  n752 = flat-sequence {
                    tunnel: w1649 -> [w1660]
                    tunnel: [w1676] -> w1646
                    tunnel: w1642 -> [w1675]
                    tunnel: w1641 -> [w1674]
                    tunnel: [w1663] -> w1639
                    tunnel: [w1662] -> w1643
                    frame #0 {
                      n753 = for {
                        tunnel: w1660 -> [w1724] mode=indexing
                        tunnel: [w1717] -> w1680 mode=indexing
                        tunnel: w1675 -> [w1712]
                        tunnel: w1674 -> [w1713]
                        n754 = call-poly <vilib>:"Basic Averaged DC-RMS.vi"("signal in"=w1724) -> ("DC value"=w1725:dbl)  [unwired: 7 in, 3 out]
                        n755 = Subtract(x=w1724, y=w1725) -> (x-y=w1714:dbl[])
                        n756 = Divide(x=w1712, y=w1713) -> (x/y=w1721:dbl)
                        n757 = Array Size(array=w1714) -> (size(s)=w1722:i32)
                        n758 = Subtract(x=w1722, y=w1721) -> (x-y=w1723:dbl)
                        n759 = for {
                          N: w1723 -> [_]
                          tunnel: w1721 -> [w1727]
                          tunnel: [w1730] -> w1715 mode=indexing
                          tunnel: w1714 -> [w1729]
                          i -> [w1728]
                          n760 = Array Subset(array=w1729, index=w1728, length=w1727) -> (w1726:dbl[])
                          n761 = call-poly <vilib>:"RMS.vi"("X"=w1726) -> ("rms value"=w1730:dbl)  [unwired: 1 out]
                        }
                        n762 = Array Max & Min(array=w1715) -> (max value=w1719:dbl, min value=w1718:dbl)  [unwired: 2 out]
                        n763 = call <vilib>:"Std Deviation and Variance.vi"("X"=w1715) -> ("mean"=w1716:dbl)  [unwired: 1 in, 2 out]
                        n764 = call <vilib>:"Median.vi"("X"=w1715) -> ("median"=w1720:dbl)  [unwired: 1 out]
                        n765 = Build Array(w1716, w1720, w1719, w1718) -> (w1717:dbl[])
                      }
                      n766 = Multiply(x=w1680, y=1000 ("median")) -> (x*y=w1659:dbl[][])
                      n767 = Index Array(array=w1659, index (col) #1=0 ("disabled index (col)"), index (col) #2=1 ("index (col)"), index (col) #3=2 ("index (col)"), index (col) #4=3 ("index (col)")) -> (element #1=→"mean":dbl[], element #2=→"median":dbl[], element #3=→"max":dbl[], element #4=→"min":dbl[])  [unwired: 4 in]
                      n768 = for {
                        tunnel: w1659 -> [w1707] mode=indexing
                        tunnel: [w1704] -> w1661 mode=indexing
                        tunnel: [w1702] -> w1650 mode=indexing
                        (unwired) 0.2 ("x")
                        n769 = local read "noise_range"() -> (w1703:dbl)
                        n770 = call <vilib>:"Median.vi"("X"=w1707) -> ("median"=w1702:dbl)  [unwired: 1 out]
                        n771 = Subtract(x=w1702, y=w1703) -> (x-y=w1705:dbl)
                        n772 = Add(x=w1703, y=w1702) -> (x+y=w1706:dbl)
                        n773 = for {
                          tunnel: w1707 -> [w1711] mode=indexing
                          tunnel: w1706 -> [w1710]
                          tunnel: w1705 -> [w1709]
                          tunnel: [w1708] -> w1704 mode=indexing
                          n774 = In Range and Coerce(upper limit=w1710, x=w1711, lower limit=w1709) -> (In Range?=w1708:bool)  [unwired: 1 out]
                        }
                      }
                      "Value to compare" <- w1650
                      n775 = for {
                        tunnel: w1661 -> [w1701] mode=indexing
                        tunnel: [w1700] -> w1677 mode=indexing
                        n776 = And Array Elements(Boolean array=w1701) -> (logical AND=w1700:bool)
                      }
                      n777 = for {
                        shift-right: [w1687] -> w1676
                        shift-left: w1660 -> [w1688]
                        tunnel: w1677 -> [w1686] mode=indexing
                        shift-right: [w1683] -> w1673
                        shift-left: 0 ("index of element") -> [w1684]
                        shift-right: [w1681] -> w1668
                        shift-left: 0 ("index of element") -> [w1682]
                        i -> [w1685]
                        n778 = case shown="False" w1686 {
                          tunnel: w1688 -> [w1695 w1699]
                          tunnel: [w1694 w1699] -> w1687
                          tunnel: w1685 -> [w1693 _]
                          tunnel: w1684 -> [w1692 w1698]
                          tunnel: [w1691 w1698] -> w1683
                          tunnel: w1682 -> [w1689 w1697]
                          tunnel: [w1689 w1696] -> w1681
                          frame False {
                            n779 = Subtract(x=w1693, y=w1692) -> (x-y=w1690:i32)
                            n780 = Delete From Array(array=w1695, index (row)=w1690) -> (array with subset deleted=w1694:sgl[][])  [unwired: 2 in, 1 out]
                            n781 = Increment(x=w1692) -> (x+1=w1691:i32)
                          }
                          frame True {
                            n782 = Increment(x=w1697) -> (x+1=w1696:i32)
                          }
                        }
                      }
                      n783 = Number To Decimal String(number=w1673) -> (decimal integer string=w1671:string)  [unwired: 1 in]
                      n784 = Greater?(x=w1668, y=3) -> (0:w1662:bool)
                      n785 = Select(t="------------------------------------------------------------------------", s=w1662, f="There are not enough correct measurements to calibrate\n\nREPEAT THE ACCELEROMETER CALIBRATION\n------------------------------------------------------------------------") -> (s? t:f=w1664:string)
                      n786 = Concatenate Strings("SIGNAL NOISE ANALYSIS:\n\nFiles erasing by  noise: ", w1671, "\r", w1664) -> (w1663:string)
                    }
                  }
                  n787 = local read "Report"() -> (w1644:string)
                  n788 = Concatenate Strings(w1639, w1644) -> (w1645:string)
                  n789 = local write "Report"(w1645) -> ()
                }
                frame "Acel_result" {
                  n790 = local read "Frecuencia de muestreo (Hz)"() -> (w1742:dbl)
                  n791 = local read "Pattern frequency (Hz)"() -> (w1741:dbl)
                  n792 = local read "Pattern amplitude (g)"() -> (w1740:dbl)
                  n793 = flat-sequence {
                    tunnel: w1743 -> [w1761]
                    tunnel: w1742 -> [w1759]
                    tunnel: w1741 -> [w1758]
                    tunnel: w1740 -> [w1757]
                    tunnel: [w1756] -> w1736
                    tunnel: [w1747] -> _
                    tunnel: [w1746] -> w1731
                    frame #0 {
                      n794 = for {
                        tunnel: w1761 -> [w1775] mode=indexing
                        tunnel: w1759 -> [w1771]
                        tunnel: w1758 -> [w1768]
                        tunnel: [w1769] -> w1766 mode=indexing
                        n795 = call-poly <vilib>:"Basic Averaged DC-RMS.vi"("signal in"=w1775) -> ("DC value"=w1776:dbl)  [unwired: 7 in, 3 out]
                        n796 = Subtract(x=w1775, y=w1776) -> (x-y=w1767:dbl[])
                        n797 = Divide(x=w1771, y=w1768) -> (x/y=w1772:dbl)
                        n798 = Array Size(array=w1767) -> (size(s)=w1773:i32)
                        n799 = Subtract(x=w1773, y=w1772) -> (x-y=w1774:dbl)
                        n800 = for {
                          N: w1774 -> [_]
                          tunnel: w1772 -> [w1778]
                          tunnel: [w1781] -> w1770 mode=indexing
                          tunnel: w1767 -> [w1780]
                          i -> [w1779]
                          n801 = Array Subset(array=w1780, index=w1779, length=w1778) -> (w1777:dbl[])
                          n802 = call-poly <vilib>:"RMS.vi"("X"=w1777) -> ("rms value"=w1781:dbl)  [unwired: 1 out]
                        }
                        n803 = call <vilib>:"Std Deviation and Variance.vi"("X"=w1770) -> ("mean"=w1769:dbl)  [unwired: 1 in, 2 out]
                      }
                      n804 = call <vilib>:"Std Deviation and Variance.vi"("X"=w1766) -> ("mean"=w1765:dbl)  [unwired: 1 in, 2 out]
                      n805 = Divide(x=w1757, y=w1765) -> (x/y=w1763:dbl)
                      n806 = Reciprocal(x=w1763) -> (1/x=w1760:dbl)
                      n807 = Multiply(x=w1760, y=1000.0) -> (x*y=w1753:dbl)
                      n808 = Number To Fractional String(number=w1753, precision (6)=i16 2) -> (F-format string=w1749:string)  [unwired: 2 in]
                      n809 = Divide(x=w1760, y=9.81) -> (x/y=w1756:dbl)
                      n810 = In Range and Coerce(upper limit=14.5, x=w1753, lower limit=7.5) -> (In Range?=w1747:bool)  [unwired: 1 out]
                      n811 = Select(t="\n\nACCELEROMETER CALIBRATED CORRECTLY\n------------------------------------------------------------------------ \n", s=w1747, f="\n\nCALIBRATION FAILED\nSENSITIVITY OUT OF RANGE (7,5-14,5)\n------------------------------------------------------------------------ \n") -> (s? t:f=w1748:string)
                      n812 = Concatenate Strings("\nAMPLITUDE CALIBRATION:\n\nSENSIVITY: ", w1749, w1748, "\r") -> (w1746:string)
                    }
                  }
                  n813 = local read "Report"() -> (w1739:string)
                  n814 = Concatenate Strings(w1731, w1739) -> (w1738:string)
                  n815 = local write "Report"(w1738) -> ()
                  "Calibration parameter" <- w1736
                }
              }
              n816 = Wait Until Next ms Multiple(millisecond multiple=u32 200 ("milliseconds to wait")) -> ()  [unwired: 1 out]
              n817 = Not(x=w1030) -> (.not. x?=w1036:bool)
              n818 = Concatenate Strings(w1032, w1034) -> (w1033:string)
              "Numeric" <- w1031
            }
            n819 = while {
              tunnel: [w1007] -> w987
              tunnel: w988 -> [w1007]
              i -> [w1004]
              stop <- w1005 stop-if-true
              n820 = Wait (ms)(milliseconds to wait=u32 1000) -> ()  [unwired: 1 out]
              n821 = Greater?(x=w1004, y=2) -> (0:w1005:bool)
            }
            n822 = local read "calibration log"() -> (w994:path)
            n823 = Write to Text File(file (use dialog)=w994, text=w987) -> ()  [unwired: 2 in, 3 out]
            n824 = flat-sequence {
              tunnel: w993 -> [w1016]
              tunnel: w989 -> [w1015]
              tunnel: [w1016] -> w992
              tunnel: [w1015] -> w990
              frame #0 {
                # "Antes Accel. detected"
                n825 = local read "Accelerometer"() -> (w1013:i32)
                n826 = local read "Save calibration"() -> (w1012:bool)
                n827 = Add(x=w1013, y=7) -> (x+y=w1010:i32)
                n828 = Less Or Equal?(x=w1010, y=15) -> (x <= y?=w1011:bool)
                n829 = And(x=w1011, y=w1012) -> (x .and. y?=w1008:bool)
                n830 = case shown="True" w1008 {
                  tunnel: w1010 -> [_ w1017]
                  frame False {
                  }
                  frame True {
                    w1027 = "Parametros"  # Key 1
                    n831 = local read "configuration file path"() -> (w1019:path)
                    n832 = local read "Calibration parameter"() -> (w1018:dbl)
                    n833 = Number To Decimal String(number=w1017) -> (decimal integer string=w1028:string)  [unwired: 1 in]
                    n834 = Concatenate Strings(w1027, w1028) -> (w1021:string)
                    n835 = call <vilib>:"Open Config Data.vi"("create file if necessary (T)"=TRUE, "configuration file path"=w1019) -> ("error out"=w1022:errorcluster, "refnum"=w1023:T12)  [unwired: 1 in, 7 out]
                    n836 = call-poly <vilib>:"Write Key.vi"("section"="Adquisicion", "error in (no error)"=w1022, "value"=w1018, "key"=w1021, "refnum"=w1023) -> ("error out"=w1026:errorcluster, "refnum out"=w1025:T12)  [unwired: 3 in, 2 out]
                    n837 = call <vilib>:"Close Config Data.vi"("error in (no error)"=w1026, "refnum"=w1025) -> ()  [unwired: 8 in, 2 out]
                  }
                }
              }
            }
          }
          frame "UPS" {
            n838 = node-c288() -> (w1795:T6)  [unwired: 4 in]
            n839 = timed-loop {
              timing: w1795 -> [_]
              timing-out: [_] -> w1794
              tunnel: w1793 -> [w1804]
              tunnel: w1792 -> [w1803]
              tunnel: [w1802] -> w1791
              tunnel: [w1801] -> w1790
              stop <- w1796 stop-if-true
              n840 = node-c288() -> ()  [unwired: 1 in, 1 out]
              n841 = xnode "Read/Write Control"("FPGA VI Reference In"=w1804, "error in"=w1803) -> ("FPGA VI Reference Out"=w1802:refnum<k20>, "error out"=w1801:errorcluster, "DC OK"=w1799:bool, "Chassis Temperature"=w1800:i16)
              n842 = call "ControlTemperatura.vi"("Chassis Temperature"=w1800) -> ("T fuera rango"=w1798:bool)  [unwired: 2 out]
              n843 = Not(x=w1798) -> (.not. x?=w1797:bool)
              n844 = And(x=w1799, y=w1797) -> (x .and. y?=w1796:bool)
              n845 = node-c288() -> ()  [unwired: 1 in, 1 out]
            }
            n846 = node-c288(w1794) -> ()  [unwired: 1 out]
          }
        }
        "error manipulacion archivos" <- w110
        n847 = local read "Parar la aplicación"() -> (w108:bool)
      }
      n848 = case shown="True" w81 {
        frame False {
        }
        frame True {
          w89 = T13 {"IP"="169.254.1.1", "Port"=5084, "ReaderConfigFile"=path "", "ROspecConfigFile"=path ""}  # RFID Configuration
          w93 = path "" ("ReaderConfigFile")
          # "Loop RFID reader"
          n849 = local read "Puerto RFID"() -> (w91:u16)
          n850 = local read "IP RFID"() -> (w92:string)
          n851 = Bundle By Name(cluster=w89, "IP"=w92, "Port"=w91, "ReaderConfigFile"=w93, "ROspecConfigFile"=w93) -> (w90:T13)
          n852 = while {
            tunnel: w90 -> [w95]
            stop <- w96 stop-if-true
            n853 = local read "Parar la aplicación"() -> (w96:bool)
            n854 = call "IF2_Reader.vi"("Stop"=w96, "RFID Configuration"=w95) -> ("error out"=w97:errorcluster, "connection ID"=→"connection ID":refnum<k5>)  [unwired: 8 in]
            n855 = case shown="No Error" w97 {
              tunnel: w97 -> [_ w99]
              tunnel: [TRUE ("RFIDStatus") FALSE ("RFIDStatus")] -> _
              frame No Error {
              }
              frame Error {
                n856 = call "Reporting_error.vi"("error out 2"=w99, "Concept"="Passive RFID") -> ("Reporting"=w101:string)  [unwired: 1 in]
                n857 = local read "Report"() -> (w102:string)
                n858 = Concatenate Strings(w101, w102) -> (w100:string)
                n859 = local write "Report"(w100) -> ()
              }
            }
          }
        }
      }
      n860 = xnode "Close FPGA VI Reference"("FPGA VI Reference In"=w84, "error in"=w83) -> ("error out"=→"error FPGA":errorcluster)
    }
    frame #3 {
      n861 = call "LH6HD.vi"("Action"=enum16{"Init", "Start", "Read", "Stop", "Exit"}."Stop") -> ("error out"=→"RFID_LR6_Error":errorcluster)  [unwired: 9 in, 1 out]
    }
  }
